vi "Grid_multiGrid.vi"() -> ()   [LabVIEW 2014]
uses:
  <userlib>/Nanonis Prog Interface V5/Nanonis Prog Interface.lvlib
panel:
  out "size(s) 5":i32
  out "size(s) 4":i32
  out "size(s) 3":i32=11
  out "size(s) 2":i32=12
  out "size(s)":i32=15
  out "data\n\n 5":T1(array[cluster])=[{"Amplitude (mod. signal unit)"=0.0, "Lockin on/off status"=FALSE, "Backward sweep"=TRUE, "Number of points"=215, "Channels"=["Current (A)", "LI Demod 1 X (A)", "LI Demod 1 Y (A)", "LI Demod 2 X (A)", "LI Demod 2 Y (A)"], "Parameters"=["X (m)", "Y (m)", "Z (m)", "Z offset (m)", "Settling time (s)", "Integration time (s)", "Z-Ctrl hold", "Final Z (m)"], "Fixed parameters"=["Sweep Start", "Sweep End"], "Multiple sweeps configuration"={"Number of Sweeps"=1, "Save all"=FALSE}, "Initialization"={"Z averaging time (s)"=0.001, "Initial settling time (s)"=0.0002}, "Sweep Timing"={"Max. slew rate (V/s)"=inf, "Settling time (s)"=0.001, "Integration time (s)"=0.001}, "End of Sweep"={"End settling time (s)"=5e-05, "Z control time (s)"=0.0002}, "Initial Z-Offset (m)"=0.0, "Sweep Distance (m)"=0.0, "Channels 2"=[], "Name"="", "Reset Z"=FALSE, "Record final Z"=FALSE, "Auto Retract Status"=FALSE, "Threshold"=0.0, "Auto Retract Signal Index"=0, "Auto Retract Condition"=FALSE}, {"Amplitude (mod. signal unit)"=0.0, "Lockin on/off status"=FALSE, "Backward sweep"=FALSE, "Number of points"=0, "Channels"=[], "Parameters"=[], "Fixed parameters"=[], "Multiple sweeps configuration"={"Number of Sweeps"=0, "Save all"=FALSE}, "Initialization"={"Z averaging time (s)"=0.0, "Initial settling time (s)"=0.0}, "Sweep Timing"={"Max. slew rate (V/s)"=0.0, "Settling time (s)"=0.0, "Integration time (s)"=0.0}, "End of Sweep"={"End settling time (s)"=0.0, "Z control time (s)"=0.0}, "Initial Z-Offset (m)"=0.0, "Sweep Distance (m)"=0.0, "Channels 2"=[], "Name"="", "Reset Z"=FALSE, "Record final Z"=FALSE, "Auto Retract Status"=FALSE, "Threshold"=0.0, "Auto Retract Signal Index"=0, "Auto Retract Condition"=FALSE}, {"Amplitude (mod. signal unit)"=0.0, "Lockin on/off status"=FALSE, "Backward sweep"=FALSE, "Number of points"=0, "Channels"=[], "Parameters"=[], "Fixed parameters"=[], "Multiple sweeps configuration"={"Number of Sweeps"=0, "Save all"=FALSE}, "Initialization"={"Z averaging time (s)"=0.0, "Initial settling time (s)"=0.0}, "Sweep Timing"={"Max. slew rate (V/s)"=0.0, "Settling time (s)"=0.0, "Integration time (s)"=0.0}, "End of Sweep"={"End settling time (s)"=0.0, "Z control time (s)"=0.0}, "Initial Z-Offset (m)"=0.0, "Sweep Distance (m)"=0.0, "Channels 2"=[], "Name"="", "Reset Z"=FALSE, "Record final Z"=FALSE, "Auto Retract Status"=FALSE, "Threshold"=0.0, "Auto Retract Signal Index"=0, "Auto Retract Condition"=FALSE}, {"Amplitude (mod. signal unit)"=0.0, "Lockin on/off status"=FALSE, "Backward sweep"=FALSE, "Number of points"=0, "Channels"=[], "Parameters"=[], "Fixed parameters"=[], "Multiple sweeps configuration"={"Number of Sweeps"=0, "Save all"=FALSE}, "Initialization"={"Z averaging time (s)"=0.0, "Initial settling time (s)"=0.0}, "Sweep Timing"={"Max. slew rate (V/s)"=0.0, "Settling time (s)"=0.0, "Integration time (s)"=0.0}, "End of Sweep"={"End settling time (s)"=0.0, "Z control time (s)"=0.0}, "Initial Z-Offset (m)"=0.0, "Sweep Distance (m)"=0.0, "Channels 2"=[], "Name"="", "Reset Z"=FALSE, "Record final Z"=FALSE, "Auto Retract Status"=FALSE, "Threshold"=0.0, "Auto Retract Signal Index"=0, "Auto Retract Condition"=FALSE}, {"Amplitude (mod. signal unit)"=0.0, "Lockin on/off status"=FALSE, "Backward sweep"=FALSE, "Number of points"=0, "Channels"=[], "Parameters"=[], "Fixed parameters"=[], "Multiple sweeps configuration"={"Number of Sweeps"=0, "Save all"=FALSE}, "Initialization"={"Z averaging time (s)"=0.0, "Initial settling time (s)"=0.0}, "Sweep Timing"={"Max. slew rate (V/s)"=0.0, "Settling time (s)"=0.0, "Integration time (s)"=0.0}, "End of Sweep"={"End settling time (s)"=0.0, "Z control time (s)"=0.0}, "Initial Z-Offset (m)"=0.0, "Sweep Distance (m)"=0.0, "Channels 2"=[], "Name"="", "Reset Z"=FALSE, "Record final Z"=FALSE, "Auto Retract Status"=FALSE, "Threshold"=0.0, "Auto Retract Signal Index"=0, "Auto Retract Condition"=FALSE}, {"Amplitude (mod. signal unit)"=0.0, "Lockin on/off status"=FALSE, "Backward sweep"=FALSE, "Number of points"=0, "Channels"=[], "Parameters"=[], "Fixed parameters"=[], "Multiple sweeps configuration"={"Number of Sweeps"=0, "Save all"=FALSE}, "Initialization"={"Z averaging time (s)"=0.0, "Initial settling time (s)"=0.0}, "Sweep Timing"={"Max. slew rate (V/s)"=0.0, "Settling time (s)"=0.0, "Integration time (s)"=0.0}, "End of Sweep"={"End settling time (s)"=0.0, "Z control time (s)"=0.0}, "Initial Z-Offset (m)"=0.0, "Sweep Distance (m)"=0.0, "Channels 2"=[], "Name"="", "Reset Z"=FALSE, "Record final Z"=FALSE, "Auto Retract Status"=FALSE, "Threshold"=0.0, "Auto Retract Signal Index"=0, "Auto Retract Condition"=FALSE}, {"Amplitude (mod. signal unit)"=0.0, "Lockin on/off status"=FALSE, "Backward sweep"=FALSE, "Number of points"=0, "Channels"=[], "Parameters"=[], "Fixed parameters"=[], "Multiple sweeps configuration"={"Number of Sweeps"=0, "Save all"=FALSE}, "Initialization"={"Z averaging time (s)"=0.0, "Initial settling time (s)"=0.0}, "Sweep Timing"={"Max. slew rate (V/s)"=0.0, "Settling time (s)"=0.0, "Integration time (s)"=0.0}, "End of Sweep"={"End settling time (s)"=0.0, "Z control time (s)"=0.0}, "Initial Z-Offset (m)"=0.0, "Sweep Distance (m)"=0.0, "Channels 2"=[], "Name"="", "Reset Z"=FALSE, "Record final Z"=FALSE, "Auto Retract Status"=FALSE, "Threshold"=0.0, "Auto Retract Signal Index"=0, "Auto Retract Condition"=FALSE}, {"Amplitude (mod. signal unit)"=0.0, "Lockin on/off status"=FALSE, "Backward sweep"=FALSE, "Number of points"=0, "Channels"=[], "Parameters"=[], "Fixed parameters"=[], "Multiple sweeps configuration"={"Number of Sweeps"=0, "Save all"=FALSE}, "Initialization"={"Z averaging time (s)"=0.0, "Initial settling time (s)"=0.0}, "Sweep Timing"={"Max. slew rate (V/s)"=0.0, "Settling time (s)"=0.0, "Integration time (s)"=0.0}, "End of Sweep"={"End settling time (s)"=0.0, "Z control time (s)"=0.0}, "Initial Z-Offset (m)"=0.0, "Sweep Distance (m)"=0.0, "Channels 2"=[], "Name"="", "Reset Z"=FALSE, "Record final Z"=FALSE, "Auto Retract Status"=FALSE, "Threshold"=0.0, "Auto Retract Signal Index"=0, "Auto Retract Condition"=FALSE}, {"Amplitude (mod. signal unit)"=0.0, "Lockin on/off status"=FALSE, "Backward sweep"=FALSE, "Number of points"=0, "Channels"=[], "Parameters"=[], "Fixed parameters"=[], "Multiple sweeps configuration"={"Number of Sweeps"=0, "Save all"=FALSE}, "Initialization"={"Z averaging time (s)"=0.0, "Initial settling time (s)"=0.0}, "Sweep Timing"={"Max. slew rate (V/s)"=0.0, "Settling time (s)"=0.0, "Integration time (s)"=0.0}, "End of Sweep"={"End settling time (s)"=0.0, "Z control time (s)"=0.0}, "Initial Z-Offset (m)"=0.0, "Sweep Distance (m)"=0.0, "Channels 2"=[], "Name"="", "Reset Z"=FALSE, "Record final Z"=FALSE, "Auto Retract Status"=FALSE, "Threshold"=0.0, "Auto Retract Signal Index"=0, "Auto Retract Condition"=FALSE}, {"Amplitude (mod. signal unit)"=0.0, "Lockin on/off status"=FALSE, "Backward sweep"=FALSE, "Number of points"=0, "Channels"=[], "Parameters"=[], "Fixed parameters"=[], "Multiple sweeps configuration"={"Number of Sweeps"=0, "Save all"=FALSE}, "Initialization"={"Z averaging time (s)"=0.0, "Initial settling time (s)"=0.0}, "Sweep Timing"={"Max. slew rate (V/s)"=0.0, "Settling time (s)"=0.0, "Integration time (s)"=0.0}, "End of Sweep"={"End settling time (s)"=0.0, "Z control time (s)"=0.0}, "Initial Z-Offset (m)"=0.0, "Sweep Distance (m)"=0.0, "Channels 2"=[], "Name"="", "Reset Z"=FALSE, "Record final Z"=FALSE, "Auto Retract Status"=FALSE, "Threshold"=0.0, "Auto Retract Signal Index"=0, "Auto Retract Condition"=FALSE}, {"Amplitude (mod. signal unit)"=0.0, "Lockin on/off status"=FALSE, "Backward sweep"=FALSE, "Number of points"=0, "Channels"=[], "Parameters"=[], "Fixed parameters"=[], "Multiple sweeps configuration"={"Number of Sweeps"=0, "Save all"=FALSE}, "Initialization"={"Z averaging time (s)"=0.0, "Initial settling time (s)"=0.0}, "Sweep Timing"={"Max. slew rate (V/s)"=0.0, "Settling time (s)"=0.0, "Integration time (s)"=0.0}, "End of Sweep"={"End settling time (s)"=0.0, "Z control time (s)"=0.0}, "Initial Z-Offset (m)"=0.0, "Sweep Distance (m)"=0.0, "Channels 2"=[], "Name"="", "Reset Z"=FALSE, "Record final Z"=FALSE, "Auto Retract Status"=FALSE, "Threshold"=0.0, "Auto Retract Signal Index"=0, "Auto Retract Condition"=FALSE}, {"Amplitude (mod. signal unit)"=0.0, "Lockin on/off status"=FALSE, "Backward sweep"=FALSE, "Number of points"=0, "Channels"=[], "Parameters"=[], "Fixed parameters"=[], "Multiple sweeps configuration"={"Number of Sweeps"=0, "Save all"=FALSE}, "Initialization"={"Z averaging time (s)"=0.0, "Initial settling time (s)"=0.0}, "Sweep Timing"={"Max. slew rate (V/s)"=0.0, "Settling time (s)"=0.0, "Integration time (s)"=0.0}, "End of Sweep"={"End settling time (s)"=0.0, "Z control time (s)"=0.0}, "Initial Z-Offset (m)"=0.0, "Sweep Distance (m)"=0.0, "Channels 2"=[], "Name"="", "Reset Z"=FALSE, "Record final Z"=FALSE, "Auto Retract Status"=FALSE, "Threshold"=0.0, "Auto Retract Signal Index"=0, "Auto Retract Condition"=FALSE}, {"Amplitude (mod. signal unit)"=0.0, "Lockin on/off status"=FALSE, "Backward sweep"=FALSE, "Number of points"=0, "Channels"=[], "Parameters"=[], "Fixed parameters"=[], "Multiple sweeps configuration"={"Number of Sweeps"=0, "Save all"=FALSE}, "Initialization"={"Z averaging time (s)"=0.0, "Initial settling time (s)"=0.0}, "Sweep Timing"={"Max. slew rate (V/s)"=0.0, "Settling time (s)"=0.0, "Integration time (s)"=0.0}, "End of Sweep"={"End settling time (s)"=0.0, "Z control time (s)"=0.0}, "Initial Z-Offset (m)"=0.0, "Sweep Distance (m)"=0.0, "Channels 2"=[], "Name"="", "Reset Z"=FALSE, "Record final Z"=FALSE, "Auto Retract Status"=FALSE, "Threshold"=0.0, "Auto Retract Signal Index"=0, "Auto Retract Condition"=FALSE}, {"Amplitude (mod. signal unit)"=0.0, "Lockin on/off status"=FALSE, "Backward sweep"=FALSE, "Number of points"=0, "Channels"=[], "Parameters"=[], "Fixed parameters"=[], "Multiple sweeps configuration"={"Number of Sweeps"=0, "Save all"=FALSE}, "Initialization"={"Z averaging time (s)"=0.0, "Initial settling time (s)"=0.0}, "Sweep Timing"={"Max. slew rate (V/s)"=0.0, "Settling time (s)"=0.0, "Integration time (s)"=0.0}, "End of Sweep"={"End settling time (s)"=0.0, "Z control time (s)"=0.0}, "Initial Z-Offset (m)"=0.0, "Sweep Distance (m)"=0.0, "Channels 2"=[], "Name"="", "Reset Z"=FALSE, "Record final Z"=FALSE, "Auto Retract Status"=FALSE, "Threshold"=0.0, "Auto Retract Signal Index"=0, "Auto Retract Condition"=FALSE}, {"Amplitude (mod. signal unit)"=0.0, "Lockin on/off status"=FALSE, "Backward sweep"=FALSE, "Number of points"=0, "Channels"=[], "Parameters"=[], "Fixed parameters"=[], "Multiple sweeps configuration"={"Number of Sweeps"=0, "Save all"=FALSE}, "Initialization"={"Z averaging time (s)"=0.0, "Initial settling time (s)"=0.0}, "Sweep Timing"={"Max. slew rate (V/s)"=0.0, "Settling time (s)"=0.0, "Integration time (s)"=0.0}, "End of Sweep"={"End settling time (s)"=0.0, "Z control time (s)"=0.0}, "Initial Z-Offset (m)"=0.0, "Sweep Distance (m)"=0.0, "Channels 2"=[], "Name"="", "Reset Z"=FALSE, "Record final Z"=FALSE, "Auto Retract Status"=FALSE, "Threshold"=0.0, "Auto Retract Signal Index"=0, "Auto Retract Condition"=FALSE}, {"Amplitude (mod. signal unit)"=0.0, "Lockin on/off status"=FALSE, "Backward sweep"=FALSE, "Number of points"=0, "Channels"=[], "Parameters"=[], "Fixed parameters"=[], "Multiple sweeps configuration"={"Number of Sweeps"=0, "Save all"=FALSE}, "Initialization"={"Z averaging time (s)"=0.0, "Initial settling time (s)"=0.0}, "Sweep Timing"={"Max. slew rate (V/s)"=0.0, "Settling time (s)"=0.0, "Integration time (s)"=0.0}, "End of Sweep"={"End settling time (s)"=0.0, "Z control time (s)"=0.0}, "Initial Z-Offset (m)"=0.0, "Sweep Distance (m)"=0.0, "Channels 2"=[], "Name"="", "Reset Z"=FALSE, "Record final Z"=FALSE, "Auto Retract Status"=FALSE, "Threshold"=0.0, "Auto Retract Signal Index"=0, "Auto Retract Condition"=FALSE}, {"Amplitude (mod. signal unit)"=0.0, "Lockin on/off status"=FALSE, "Backward sweep"=FALSE, "Number of points"=0, "Channels"=[], "Parameters"=[], "Fixed parameters"=[], "Multiple sweeps configuration"={"Number of Sweeps"=0, "Save all"=FALSE}, "Initialization"={"Z averaging time (s)"=0.0, "Initial settling time (s)"=0.0}, "Sweep Timing"={"Max. slew rate (V/s)"=0.0, "Settling time (s)"=0.0, "Integration time (s)"=0.0}, "End of Sweep"={"End settling time (s)"=0.0, "Z control time (s)"=0.0}, "Initial Z-Offset (m)"=0.0, "Sweep Distance (m)"=0.0, "Channels 2"=[], "Name"="", "Reset Z"=FALSE, "Record final Z"=FALSE, "Auto Retract Status"=FALSE, "Threshold"=0.0, "Auto Retract Signal Index"=0, "Auto Retract Condition"=FALSE}, {"Amplitude (mod. signal unit)"=0.0, "Lockin on/off status"=FALSE, "Backward sweep"=FALSE, "Number of points"=0, "Channels"=[], "Parameters"=[], "Fixed parameters"=[], "Multiple sweeps configuration"={"Number of Sweeps"=0, "Save all"=FALSE}, "Initialization"={"Z averaging time (s)"=0.0, "Initial settling time (s)"=0.0}, "Sweep Timing"={"Max. slew rate (V/s)"=0.0, "Settling time (s)"=0.0, "Integration time (s)"=0.0}, "End of Sweep"={"End settling time (s)"=0.0, "Z control time (s)"=0.0}, "Initial Z-Offset (m)"=0.0, "Sweep Distance (m)"=0.0, "Channels 2"=[], "Name"="", "Reset Z"=FALSE, "Record final Z"=FALSE, "Auto Retract Status"=FALSE, "Threshold"=0.0, "Auto Retract Signal Index"=0, "Auto Retract Condition"=FALSE}]
  out "data\n\n 2":T2(array[cluster])=[{"Amplitude (mod. signal unit)"=0.0, "Lockin on/off status"=FALSE, "Advanced options"={"Z-Controller Hold"=TRUE, "Record final Z"=FALSE, "Reset Bias"=TRUE}, "Backward sweep"=TRUE, "Number of points"=215, "Channels"=["Current (A)", "LI Demod 1 X (A)", "LI Demod 1 Y (A)", "LI Demod 2 X (A)", "LI Demod 2 Y (A)"], "Parameters"=["X (m)", "Y (m)", "Z (m)", "Z offset (m)", "Settling time (s)", "Integration time (s)", "Z-Ctrl hold", "Final Z (m)"], "Fixed parameters"=["Sweep Start", "Sweep End"], "Multiple sweeps configuration"={"Number of Sweeps"=1, "Save all"=FALSE}, "Initialization"={"Z averaging time (s)"=0.001, "Z offset (m)"=0.0, "Initial settling time (s)"=0.0002}, "Sweep Timing"={"Max. slew rate (V/s)"=inf, "Settling time (s)"=0.001, "Integration time (s)"=0.001}, "End of Sweep"={"End settling time (s)"=5e-05, "Z control time (s)"=0.0002}, "Start value (V)"=-0.02, "End value (V)"=-3.0, "Channels 2"=[0, 20, 21, 22, 23], "Name"="numerical_DCA_-20mV->-3V"}, {"Amplitude (mod. signal unit)"=0.0, "Lockin on/off status"=FALSE, "Advanced options"={"Z-Controller Hold"=TRUE, "Record final Z"=FALSE, "Reset Bias"=TRUE}, "Backward sweep"=TRUE, "Number of points"=215, "Channels"=["Current (A)", "LI Demod 1 X (A)", "LI Demod 1 Y (A)", "LI Demod 2 X (A)", "LI Demod 2 Y (A)"], "Parameters"=["X (m)", "Y (m)", "Z (m)", "Z offset (m)", "Settling time (s)", "Integration time (s)", "Z-Ctrl hold", "Final Z (m)"], "Fixed parameters"=["Sweep Start", "Sweep End"], "Multiple sweeps configuration"={"Number of Sweeps"=1, "Save all"=FALSE}, "Initialization"={"Z averaging time (s)"=0.001, "Z offset (m)"=0.0, "Initial settling time (s)"=0.0002}, "Sweep Timing"={"Max. slew rate (V/s)"=inf, "Settling time (s)"=0.001, "Integration time (s)"=0.001}, "End of Sweep"={"End settling time (s)"=5e-05, "Z control time (s)"=0.0002}, "Start value (V)"=-0.02, "End value (V)"=0.7, "Channels 2"=[0, 20, 21, 22, 23], "Name"="numerical_DCA_-20mV->0.7V"}, {"Amplitude (mod. signal unit)"=0.0, "Lockin on/off status"=FALSE, "Advanced options"={"Z-Controller Hold"=TRUE, "Record final Z"=FALSE, "Reset Bias"=TRUE}, "Backward sweep"=TRUE, "Number of points"=215, "Channels"=["Current (A)", "LI Demod 1 X (A)", "LI Demod 1 Y (A)", "LI Demod 2 X (A)", "LI Demod 2 Y (A)"], "Parameters"=["X (m)", "Y (m)", "Z (m)", "Z offset (m)", "Settling time (s)", "Integration time (s)", "Z-Ctrl hold", "Final Z (m)"], "Fixed parameters"=["Sweep Start", "Sweep End"], "Multiple sweeps configuration"={"Number of Sweeps"=30, "Save all"=FALSE}, "Initialization"={"Z averaging time (s)"=0.001, "Z offset (m)"=0.0, "Initial settling time (s)"=0.0002}, "Sweep Timing"={"Max. slew rate (V/s)"=inf, "Settling time (s)"=0.001, "Integration time (s)"=0.001}, "End of Sweep"={"End settling time (s)"=5e-05, "Z control time (s)"=0.0002}, "Start value (V)"=-0.02, "End value (V)"=0.7, "Channels 2"=[0, 20, 21, 22, 23], "Name"="numerical_DCA_-20mV->-0.7V_30sweeps"}, {"Amplitude (mod. signal unit)"=0.0, "Lockin on/off status"=FALSE, "Advanced options"={"Z-Controller Hold"=TRUE, "Record final Z"=FALSE, "Reset Bias"=TRUE}, "Backward sweep"=TRUE, "Number of points"=215, "Channels"=["Current (A)", "LI Demod 1 X (A)", "LI Demod 1 Y (A)", "LI Demod 2 X (A)", "LI Demod 2 Y (A)"], "Parameters"=["X (m)", "Y (m)", "Z (m)", "Z offset (m)", "Settling time (s)", "Integration time (s)", "Z-Ctrl hold", "Final Z (m)"], "Fixed parameters"=["Sweep Start", "Sweep End"], "Multiple sweeps configuration"={"Number of Sweeps"=50, "Save all"=FALSE}, "Initialization"={"Z averaging time (s)"=0.001, "Z offset (m)"=0.0, "Initial settling time (s)"=0.0002}, "Sweep Timing"={"Max. slew rate (V/s)"=inf, "Settling time (s)"=0.001, "Integration time (s)"=0.001}, "End of Sweep"={"End settling time (s)"=5e-05, "Z control time (s)"=0.0002}, "Start value (V)"=-0.02, "End value (V)"=0.7, "Channels 2"=[0, 20, 21, 22, 23], "Name"="numerical_DCA_-20mV->-0.7V_50_sweeps"}, {"Amplitude (mod. signal unit)"=0.0, "Lockin on/off status"=FALSE, "Advanced options"={"Z-Controller Hold"=TRUE, "Record final Z"=FALSE, "Reset Bias"=TRUE}, "Backward sweep"=TRUE, "Number of points"=215, "Channels"=["Current (A)", "LI Demod 1 X (A)", "LI Demod 1 Y (A)", "LI Demod 2 X (A)", "LI Demod 2 Y (A)"], "Parameters"=["X (m)", "Y (m)", "Z (m)", "Z offset (m)", "Settling time (s)", "Integration time (s)", "Z-Ctrl hold", "Final Z (m)"], "Fixed parameters"=["Sweep Start", "Sweep End"], "Multiple sweeps configuration"={"Number of Sweeps"=70, "Save all"=FALSE}, "Initialization"={"Z averaging time (s)"=0.001, "Z offset (m)"=0.0, "Initial settling time (s)"=0.0002}, "Sweep Timing"={"Max. slew rate (V/s)"=inf, "Settling time (s)"=0.001, "Integration time (s)"=0.001}, "End of Sweep"={"End settling time (s)"=5e-05, "Z control time (s)"=0.0002}, "Start value (V)"=-0.02, "End value (V)"=-3.0, "Channels 2"=[0, 20, 21, 22, 23], "Name"="numerical_DCA_-20mV->-3V_70sweeps"}, {"Amplitude (mod. signal unit)"=0.0, "Lockin on/off status"=FALSE, "Advanced options"={"Z-Controller Hold"=TRUE, "Record final Z"=FALSE, "Reset Bias"=TRUE}, "Backward sweep"=TRUE, "Number of points"=215, "Channels"=["Current (A)", "LI Demod 1 X (A)", "LI Demod 1 Y (A)", "LI Demod 2 X (A)", "LI Demod 2 Y (A)"], "Parameters"=["X (m)", "Y (m)", "Z (m)", "Z offset (m)", "Settling time (s)", "Integration time (s)", "Z-Ctrl hold", "Final Z (m)"], "Fixed parameters"=["Sweep Start", "Sweep End"], "Multiple sweeps configuration"={"Number of Sweeps"=100, "Save all"=FALSE}, "Initialization"={"Z averaging time (s)"=0.001, "Z offset (m)"=0.0, "Initial settling time (s)"=0.0002}, "Sweep Timing"={"Max. slew rate (V/s)"=inf, "Settling time (s)"=0.001, "Integration time (s)"=0.001}, "End of Sweep"={"End settling time (s)"=5e-05, "Z control time (s)"=0.0002}, "Start value (V)"=-0.02, "End value (V)"=-3.0, "Channels 2"=[0, 20, 21, 22, 23], "Name"="numerical_DCA_-20mV->3V_100_sweeps"}, {"Amplitude (mod. signal unit)"=0.0, "Lockin on/off status"=FALSE, "Advanced options"={"Z-Controller Hold"=TRUE, "Record final Z"=FALSE, "Reset Bias"=TRUE}, "Backward sweep"=TRUE, "Number of points"=256, "Channels"=["Current (A)", "LI Demod 1 X (A)", "LI Demod 1 Y (A)", "LI Demod 2 X (A)", "LI Demod 2 Y (A)"], "Parameters"=["X (m)", "Y (m)", "Z (m)", "Z offset (m)", "Settling time (s)", "Integration time (s)", "Z-Ctrl hold", "Final Z (m)"], "Fixed parameters"=["Sweep Start", "Sweep End"], "Multiple sweeps configuration"={"Number of Sweeps"=100, "Save all"=FALSE}, "Initialization"={"Z averaging time (s)"=0.001, "Z offset (m)"=0.0, "Initial settling time (s)"=5e-05}, "Sweep Timing"={"Max. slew rate (V/s)"=inf, "Settling time (s)"=0.001, "Integration time (s)"=0.0005}, "End of Sweep"={"End settling time (s)"=5e-05, "Z control time (s)"=5e-05}, "Start value (V)"=-1.0, "End value (V)"=2.0, "Channels 2"=[0, 20, 21, 22, 23], "Name"="numerical_-1V->2V"}, {"Amplitude (mod. signal unit)"=0.0, "Lockin on/off status"=FALSE, "Advanced options"={"Z-Controller Hold"=TRUE, "Record final Z"=FALSE, "Reset Bias"=TRUE}, "Backward sweep"=TRUE, "Number of points"=256, "Channels"=["Current (A)", "LI Demod 1 X (A)", "LI Demod 1 Y (A)", "LI Demod 2 X (A)", "LI Demod 2 Y (A)"], "Parameters"=["X (m)", "Y (m)", "Z (m)", "Z offset (m)", "Settling time (s)", "Integration time (s)", "Z-Ctrl hold", "Final Z (m)"], "Fixed parameters"=["Sweep Start", "Sweep End"], "Multiple sweeps configuration"={"Number of Sweeps"=100, "Save all"=FALSE}, "Initialization"={"Z averaging time (s)"=0.001, "Z offset (m)"=0.0, "Initial settling time (s)"=5e-05}, "Sweep Timing"={"Max. slew rate (V/s)"=inf, "Settling time (s)"=0.001, "Integration time (s)"=0.0005}, "End of Sweep"={"End settling time (s)"=5e-05, "Z control time (s)"=5e-05}, "Start value (V)"=-0.02, "End value (V)"=0.02, "Channels 2"=[0, 20, 21, 22, 23], "Name"="numerical_-20mV->20mV"}, {"Amplitude (mod. signal unit)"=0.0, "Lockin on/off status"=FALSE, "Advanced options"={"Z-Controller Hold"=TRUE, "Record final Z"=FALSE, "Reset Bias"=TRUE}, "Backward sweep"=TRUE, "Number of points"=286, "Channels"=["Current (A)", "LI Demod 1 X (A)", "LI Demod 1 Y (A)", "LI Demod 2 X (A)", "LI Demod 2 Y (A)"], "Parameters"=["X (m)", "Y (m)", "Z (m)", "Z offset (m)", "Settling time (s)", "Integration time (s)", "Z-Ctrl hold", "Final Z (m)"], "Fixed parameters"=["Sweep Start", "Sweep End"], "Multiple sweeps configuration"={"Number of Sweeps"=50, "Save all"=FALSE}, "Initialization"={"Z averaging time (s)"=0.001, "Z offset (m)"=0.0, "Initial settling time (s)"=5e-05}, "Sweep Timing"={"Max. slew rate (V/s)"=inf, "Settling time (s)"=0.001, "Integration time (s)"=0.0005}, "End of Sweep"={"End settling time (s)"=5e-05, "Z control time (s)"=5e-05}, "Start value (V)"=-0.2, "End value (V)"=0.8, "Channels 2"=[0, 20, 21, 22, 23], "Name"="DCA_numerical_-0.2V->0.8V"}, {"Amplitude (mod. signal unit)"=0.0, "Lockin on/off status"=FALSE, "Advanced options"={"Z-Controller Hold"=TRUE, "Record final Z"=FALSE, "Reset Bias"=TRUE}, "Backward sweep"=TRUE, "Number of points"=421, "Channels"=["Current (A)", "LI Demod 1 X (A)", "LI Demod 1 Y (A)", "LI Demod 2 X (A)", "LI Demod 2 Y (A)"], "Parameters"=["X (m)", "Y (m)", "Z (m)", "Z offset (m)", "Settling time (s)", "Integration time (s)", "Z-Ctrl hold", "Final Z (m)"], "Fixed parameters"=["Sweep Start", "Sweep End"], "Multiple sweeps configuration"={"Number of Sweeps"=100, "Save all"=FALSE}, "Initialization"={"Z averaging time (s)"=0.001, "Z offset (m)"=0.0, "Initial settling time (s)"=5e-05}, "Sweep Timing"={"Max. slew rate (V/s)"=inf, "Settling time (s)"=0.001, "Integration time (s)"=0.0005}, "End of Sweep"={"End settling time (s)"=5e-05, "Z control time (s)"=5e-05}, "Start value (V)"=-2.0, "End value (V)"=2.2, "Channels 2"=[0, 20, 21, 22, 23], "Name"="numerical_-2V->2.2V"}, {"Amplitude (mod. signal unit)"=0.0, "Lockin on/off status"=FALSE, "Advanced options"={"Z-Controller Hold"=TRUE, "Record final Z"=FALSE, "Reset Bias"=TRUE}, "Backward sweep"=TRUE, "Number of points"=500, "Channels"=["Current (A)", "LI Demod 1 X (A)", "LI Demod 1 Y (A)", "LI Demod 2 X (A)", "LI Demod 2 Y (A)"], "Parameters"=["X (m)", "Y (m)", "Z (m)", "Z offset (m)", "Settling time (s)", "Integration time (s)", "Z-Ctrl hold", "Final Z (m)"], "Fixed parameters"=["Sweep Start", "Sweep End"], "Multiple sweeps configuration"={"Number of Sweeps"=20, "Save all"=FALSE}, "Initialization"={"Z averaging time (s)"=0.001, "Z offset (m)"=0.0, "Initial settling time (s)"=0.01}, "Sweep Timing"={"Max. slew rate (V/s)"=inf, "Settling time (s)"=0.001, "Integration time (s)"=0.001}, "End of Sweep"={"End settling time (s)"=0.1, "Z control time (s)"=0.001}, "Start value (V)"=-0.2, "End value (V)"=0.8, "Channels 2"=[0, 20, 21, 22, 23], "Name"="DCA_numerical2_-0.2V->0.8V"}, {"Amplitude (mod. signal unit)"=0.0015, "Lockin on/off status"=FALSE, "Advanced options"={"Z-Controller Hold"=TRUE, "Record final Z"=FALSE, "Reset Bias"=TRUE}, "Backward sweep"=TRUE, "Number of points"=80, "Channels"=["Current (A)", "LI Demod 1 X (A)", "LI Demod 1 Y (A)", "LI Demod 2 X (A)", "LI Demod 2 Y (A)"], "Parameters"=["X (m)", "Y (m)", "Z (m)", "Z offset (m)", "Settling time (s)", "Integration time (s)", "Z-Ctrl hold", "Final Z (m)"], "Fixed parameters"=["Sweep Start", "Sweep End"], "Multiple sweeps configuration"={"Number of Sweeps"=10, "Save all"=FALSE}, "Initialization"={"Z averaging time (s)"=0.001, "Z offset (m)"=0.0, "Initial settling time (s)"=0.0046}, "Sweep Timing"={"Max. slew rate (V/s)"=inf, "Settling time (s)"=0.0046, "Integration time (s)"=0.032}, "End of Sweep"={"End settling time (s)"=5e-05, "Z control time (s)"=5e-05}, "Start value (V)"=-0.02, "End value (V)"=0.02, "Channels 2"=[0, 20, 21, 22, 23], "Name"="lockin_-20mV->20mV"}, {"Amplitude (mod. signal unit)"=0.002, "Lockin on/off status"=FALSE, "Advanced options"={"Z-Controller Hold"=TRUE, "Record final Z"=FALSE, "Reset Bias"=TRUE}, "Backward sweep"=TRUE, "Number of points"=70, "Channels"=["Current (A)", "LI Demod 1 X (A)", "LI Demod 1 Y (A)", "LI Demod 2 X (A)", "LI Demod 2 Y (A)"], "Parameters"=["X (m)", "Y (m)", "Z (m)", "Z offset (m)", "Settling time (s)", "Integration time (s)", "Z-Ctrl hold", "Final Z (m)"], "Fixed parameters"=["Sweep Start", "Sweep End"], "Multiple sweeps configuration"={"Number of Sweeps"=10, "Save all"=FALSE}, "Initialization"={"Z averaging time (s)"=0.001, "Z offset (m)"=0.0, "Initial settling time (s)"=0.0046}, "Sweep Timing"={"Max. slew rate (V/s)"=inf, "Settling time (s)"=0.0046, "Integration time (s)"=0.032}, "End of Sweep"={"End settling time (s)"=5e-05, "Z control time (s)"=5e-05}, "Start value (V)"=-0.025, "End value (V)"=0.025, "Channels 2"=[0, 20, 21, 22, 23], "Name"="lockin_-25mV->25mV"}, {"Amplitude (mod. signal unit)"=0.002, "Lockin on/off status"=FALSE, "Advanced options"={"Z-Controller Hold"=TRUE, "Record final Z"=FALSE, "Reset Bias"=TRUE}, "Backward sweep"=TRUE, "Number of points"=70, "Channels"=["Current (A)", "LI Demod 1 X (A)", "LI Demod 1 Y (A)", "LI Demod 2 X (A)", "LI Demod 2 Y (A)"], "Parameters"=["X (m)", "Y (m)", "Z (m)", "Z offset (m)", "Settling time (s)", "Integration time (s)", "Z-Ctrl hold", "Final Z (m)"], "Fixed parameters"=["Sweep Start", "Sweep End"], "Multiple sweeps configuration"={"Number of Sweeps"=10, "Save all"=FALSE}, "Initialization"={"Z averaging time (s)"=0.001, "Z offset (m)"=0.0, "Initial settling time (s)"=0.0046}, "Sweep Timing"={"Max. slew rate (V/s)"=inf, "Settling time (s)"=0.0046, "Integration time (s)"=0.032}, "End of Sweep"={"End settling time (s)"=5e-05, "Z control time (s)"=5e-05}, "Start value (V)"=-0.025, "End value (V)"=0.025, "Channels 2"=[0, 20, 21, 22, 23], "Name"="test"}, {"Amplitude (mod. signal unit)"=0.0025, "Lockin on/off status"=FALSE, "Advanced options"={"Z-Controller Hold"=TRUE, "Record final Z"=FALSE, "Reset Bias"=TRUE}, "Backward sweep"=TRUE, "Number of points"=320, "Channels"=["Current (A)", "LI Demod 1 X (A)", "LI Demod 1 Y (A)", "LI Demod 2 X (A)", "LI Demod 2 Y (A)"], "Parameters"=["X (m)", "Y (m)", "Z (m)", "Z offset (m)", "Settling time (s)", "Integration time (s)", "Z-Ctrl hold", "Final Z (m)"], "Fixed parameters"=["Sweep Start", "Sweep End"], "Multiple sweeps configuration"={"Number of Sweeps"=1, "Save all"=FALSE}, "Initialization"={"Z averaging time (s)"=0.001, "Z offset (m)"=0.0, "Initial settling time (s)"=0.0046}, "Sweep Timing"={"Max. slew rate (V/s)"=inf, "Settling time (s)"=0.0046, "Integration time (s)"=0.0042}, "End of Sweep"={"End settling time (s)"=5e-05, "Z control time (s)"=5e-05}, "Start value (V)"=0.02, "End value (V)"=-0.02, "Channels 2"=[0, 20, 21, 22, 23], "Name"="lockin_highRes_20mV_-20mV"}, {"Amplitude (mod. signal unit)"=0.005, "Lockin on/off status"=FALSE, "Advanced options"={"Z-Controller Hold"=TRUE, "Record final Z"=FALSE, "Reset Bias"=TRUE}, "Backward sweep"=TRUE, "Number of points"=256, "Channels"=["Current (A)", "LI Demod 1 X (A)", "LI Demod 1 Y (A)", "LI Demod 2 X (A)", "LI Demod 2 Y (A)"], "Parameters"=["X (m)", "Y (m)", "Z (m)", "Z offset (m)", "Settling time (s)", "Integration time (s)", "Z-Ctrl hold", "Final Z (m)"], "Fixed parameters"=["Sweep Start", "Sweep End"], "Multiple sweeps configuration"={"Number of Sweeps"=2, "Save all"=FALSE}, "Initialization"={"Z averaging time (s)"=0.001, "Z offset (m)"=0.0, "Initial settling time (s)"=0.0033}, "Sweep Timing"={"Max. slew rate (V/s)"=inf, "Settling time (s)"=0.0033, "Integration time (s)"=0.0164}, "End of Sweep"={"End settling time (s)"=5e-05, "Z control time (s)"=5e-05}, "Start value (V)"=-1.0, "End value (V)"=2.0, "Channels 2"=[0, 20, 21, 22, 23], "Name"="lockin_slow"}, {"Amplitude (mod. signal unit)"=0.005, "Lockin on/off status"=FALSE, "Advanced options"={"Z-Controller Hold"=TRUE, "Record final Z"=FALSE, "Reset Bias"=TRUE}, "Backward sweep"=TRUE, "Number of points"=310, "Channels"=["Current (A)", "LI Demod 1 X (A)", "LI Demod 1 Y (A)", "LI Demod 2 X (A)", "LI Demod 2 Y (A)"], "Parameters"=["X (m)", "Y (m)", "Z (m)", "Z offset (m)", "Settling time (s)", "Integration time (s)", "Z-Ctrl hold", "Final Z (m)"], "Fixed parameters"=["Sweep Start", "Sweep End"], "Multiple sweeps configuration"={"Number of Sweeps"=2, "Save all"=FALSE}, "Initialization"={"Z averaging time (s)"=0.001, "Z offset (m)"=0.0, "Initial settling time (s)"=0.0031}, "Sweep Timing"={"Max. slew rate (V/s)"=inf, "Settling time (s)"=0.0031, "Integration time (s)"=0.0246}, "End of Sweep"={"End settling time (s)"=5e-05, "Z control time (s)"=5e-05}, "Start value (V)"=1.5, "End value (V)"=-0.05, "Channels 2"=[0, 20, 21, 22, 23], "Name"="Lock_in_DCA_1.5V->-50mV"}, {"Amplitude (mod. signal unit)"=0.005, "Lockin on/off status"=FALSE, "Advanced options"={"Z-Controller Hold"=TRUE, "Record final Z"=FALSE, "Reset Bias"=TRUE}, "Backward sweep"=TRUE, "Number of points"=401, "Channels"=["Current (A)", "Z (m)", "LI Demod 1 X (A)", "LI Demod 1 Y (A)", "LI Demod 2 X (A)", "LI Demod 2 Y (A)"], "Parameters"=["X (m)", "Y (m)", "Z (m)", "Z offset (m)", "Settling time (s)", "Integration time (s)", "Z-Ctrl hold", "Final Z (m)"], "Fixed parameters"=["Sweep Start", "Sweep End"], "Multiple sweeps configuration"={"Number of Sweeps"=1, "Save all"=FALSE}, "Initialization"={"Z averaging time (s)"=0.001, "Z offset (m)"=0.0, "Initial settling time (s)"=0.004}, "Sweep Timing"={"Max. slew rate (V/s)"=inf, "Settling time (s)"=0.02, "Integration time (s)"=0.015}, "End of Sweep"={"End settling time (s)"=5e-05, "Z control time (s)"=0.001}, "Start value (V)"=-1.0, "End value (V)"=1.0, "Channels 2"=[0, 14, 20, 21, 22, 23], "Name"="Long_MgPc_lockin_-1->1V"}, {"Amplitude (mod. signal unit)"=0.005, "Lockin on/off status"=FALSE, "Advanced options"={"Z-Controller Hold"=TRUE, "Record final Z"=FALSE, "Reset Bias"=TRUE}, "Backward sweep"=TRUE, "Number of points"=467, "Channels"=["Current (A)", "Z (m)", "LI Demod 1 X (A)", "LI Demod 1 Y (A)", "LI Demod 2 X (A)", "LI Demod 2 Y (A)"], "Parameters"=["X (m)", "Y (m)", "Z (m)", "Z offset (m)", "Settling time (s)", "Integration time (s)", "Z-Ctrl hold", "Final Z (m)"], "Fixed parameters"=["Sweep Start", "Sweep End"], "Multiple sweeps configuration"={"Number of Sweeps"=2, "Save all"=FALSE}, "Initialization"={"Z averaging time (s)"=0.001, "Z offset (m)"=0.0, "Initial settling time (s)"=0.004}, "Sweep Timing"={"Max. slew rate (V/s)"=inf, "Settling time (s)"=0.02, "Integration time (s)"=0.0246}, "End of Sweep"={"End settling time (s)"=5e-05, "Z control time (s)"=0.001}, "Start value (V)"=-2.0, "End value (V)"=1.5, "Channels 2"=[0, 14, 20, 21, 22, 23], "Name"="MgPc_long_lockin"}, {"Amplitude (mod. signal unit)"=0.008, "Lockin on/off status"=FALSE, "Advanced options"={"Z-Controller Hold"=TRUE, "Record final Z"=FALSE, "Reset Bias"=TRUE}, "Backward sweep"=TRUE, "Number of points"=256, "Channels"=["Current (A)", "LI Demod 1 X (A)", "LI Demod 1 Y (A)", "LI Demod 2 X (A)", "LI Demod 2 Y (A)"], "Parameters"=["X (m)", "Y (m)", "Z (m)", "Z offset (m)", "Settling time (s)", "Integration time (s)", "Z-Ctrl hold", "Final Z (m)"], "Fixed parameters"=["Sweep Start", "Sweep End"], "Multiple sweeps configuration"={"Number of Sweeps"=3, "Save all"=FALSE}, "Initialization"={"Z averaging time (s)"=0.001, "Z offset (m)"=0.0, "Initial settling time (s)"=0.0033}, "Sweep Timing"={"Max. slew rate (V/s)"=inf, "Settling time (s)"=0.0033, "Integration time (s)"=0.0082}, "End of Sweep"={"End settling time (s)"=5e-05, "Z control time (s)"=5e-05}, "Start value (V)"=-1.0, "End value (V)"=2.0, "Channels 2"=[0, 20, 21, 22, 23], "Name"="lockin_slow_-1_2"}, {"Amplitude (mod. signal unit)"=0.008, "Lockin on/off status"=FALSE, "Advanced options"={"Z-Controller Hold"=TRUE, "Record final Z"=FALSE, "Reset Bias"=TRUE}, "Backward sweep"=TRUE, "Number of points"=421, "Channels"=["Current (A)", "Z (m)", "LI Demod 1 X (A)", "LI Demod 1 Y (A)", "LI Demod 2 X (A)", "LI Demod 2 Y (A)"], "Parameters"=["X (m)", "Y (m)", "Z (m)", "Z offset (m)", "Settling time (s)", "Integration time (s)", "Z-Ctrl hold", "Final Z (m)"], "Fixed parameters"=["Sweep Start", "Sweep End"], "Multiple sweeps configuration"={"Number of Sweeps"=2, "Save all"=FALSE}, "Initialization"={"Z averaging time (s)"=0.001, "Z offset (m)"=0.0, "Initial settling time (s)"=5e-05}, "Sweep Timing"={"Max. slew rate (V/s)"=inf, "Settling time (s)"=0.0164, "Integration time (s)"=0.0164}, "End of Sweep"={"End settling time (s)"=5e-05, "Z control time (s)"=0.001}, "Start value (V)"=-2.0, "End value (V)"=2.2, "Channels 2"=[0, 14, 20, 21, 22, 23], "Name"="MgPc_long_lockin2"}, {"Amplitude (mod. signal unit)"=0.01, "Lockin on/off status"=FALSE, "Advanced options"={"Z-Controller Hold"=TRUE, "Record final Z"=FALSE, "Reset Bias"=TRUE}, "Backward sweep"=TRUE, "Number of points"=512, "Channels"=["Current (A)", "LI Demod 1 X (A)", "LI Demod 1 Y (A)", "LI Demod 2 X (A)", "LI Demod 2 Y (A)"], "Parameters"=["X (m)", "Y (m)", "Z (m)", "Z offset (m)", "Settling time (s)", "Integration time (s)", "Z-Ctrl hold", "Final Z (m)"], "Fixed parameters"=["Sweep Start", "Sweep End"], "Multiple sweeps configuration"={"Number of Sweeps"=1, "Save all"=FALSE}, "Initialization"={"Z averaging time (s)"=0.001, "Z offset (m)"=0.0, "Initial settling time (s)"=0.2}, "Sweep Timing"={"Max. slew rate (V/s)"=inf, "Settling time (s)"=0.0082, "Integration time (s)"=0.041}, "End of Sweep"={"End settling time (s)"=5e-05, "Z control time (s)"=5e-05}, "Start value (V)"=-3.0, "End value (V)"=2.0, "Channels 2"=[0, 20, 21, 22, 23], "Name"="Quick_Lockin"}]
  in  "Save As":string
  in  "Zspecparam.txt location":path=path "D:/Scripts/STSparam - Copy (2).txt"
  in  "Save As 2":string
  in  "STSparam.txt location":path=path "D:/Scripts/STSparam.txt"
  in  "Update STS/Zspec Param List":bool
  in  "START EXPERIMENT":bool
  in  "stop":bool
  in  "Duplicate Page 1":bool
  in  "No. of Exp":dbl=2.0 caption="No. of Experiments \n(If more than 5, edit VI)" step=1.0
  in  "Tab Control":T3(tab)=enum."Page 2"
  in  "Experiment 1":T4={"Drift Correction Settings"={"Drift Correction every"=4, "Drift correction Pixels"=128, "Channel index (0-23)"=0, "MaxImagesBack"=2, "Threshold"=2, "Increment"=1, "max applied Drift Correction"=40, "Correct Drift"=TRUE, "Correlate"=0, "Correct z drift"=FALSE, "zdrift \nDuration (s)"=0.0}, "Spectroscopy Setting"={"Imaging Current"=5e-11, "ref Current"=5e-12, "tip Speed (m/s)"=2e-09, "Imaging Bias"=-2.4, "ref Bias"=-0.02, "preSTS delay [ms]"=500, "STS z offset"=2e-10, "during Spec Bias (V)"=-0.02, "trigger1 < Hz"=0.0, "trigger 2 >Hz"=0.0, "autoStop"=FALSE, "Spectroscopy"=0, "PLL ON/OFF"=FALSE, "readjust setpoint every "=1, "z Reference"=TRUE, "Lock In"=FALSE}, "Misc"={"File name"="DCA_Zdependence_STS_Neg_Bias_Mol5_1_zOffset=200pm", "Email when finished"="Dhaneesh.Gopalakrishnan@monash.edu"}, "Grid Settings"={"type"=0, "type order"=0, "X pixel"=6, "Y pixel"=1, "Grid_Parms"={"center X (m)"=0.0, "center Y (m)"=0.0, "width (m)"=0.0, "height (m)"=0.0, "angle (deg)"=0.0}}, "STS Param List #1 "=4, "ZSpec Param List #1  "=0, "Repeat Experiment"={"Repeat"=TRUE, "Repeat Parameter"=2, "Values List #1"=14}} {"Repeat Experiment"."Repeat Parameter" items=["ref Current", "ref Bias", "STS z offset", "during Spec Bias (V)"]; "STS Param List #1" items=["numerical_DCA_-20mV->-3V", "numerical_DCA_-20mV->0.7V", "numerical_DCA_-20mV->-0.7V_30sweeps", "numerical_DCA_-20mV->-0.7V_50_sweeps", "numerical_DCA_-20mV->-3V_70sweeps", "numerical_DCA_-20mV->3V_100_sweeps", "KPFM_MgPc", "KPFM_MgPc2", "KPFM_MgPc_marina", "numerical_-1V->2V", "numerical_-20mV->20mV", "DCA_numerical_-0.2V->0.8V", "numerical_-2V->2.2V", "DCA_numerical2_-0.2V->0.8V", "lockin_-20mV->20mV", "lockin_-25mV->25mV", "test", "lockin_highRes_20mV_-20mV", "lockin_slow", "Lock_in_DCA_1.5V->-50mV", "Long_MgPc_lockin_-1->1V", "MgPc_long_lockin", "lockin_slow_-1_2", "MgPc_long_lockin2", "Quick_Lockin"]; "Grid Settings"."type order" items=["Grid", "Random", "Adam7"]; "Grid Settings"."type" items=["Line", "Grid", "Cloud"]; "Spectroscopy Setting"."Spectroscopy" items=["Bias", "zSpec"]; "Spectroscopy Setting"."trigger 2 >Hz" format="%#_6p"; "Spectroscopy Setting"."trigger1 < Hz" format="%#_6p"; "Spectroscopy Setting"."during Spec Bias (V)" format="%#_5p"; "Spectroscopy Setting"."STS z offset" format="%#_6p"; "Spectroscopy Setting"."ref Bias" format="%#_6p"; "Spectroscopy Setting"."Imaging Bias" format="%#_6p"; "Spectroscopy Setting"."tip Speed (m/s)" format="%.2p"; "Spectroscopy Setting"."ref Current" format="%#_6p"; "Spectroscopy Setting"."Imaging Current" format="%#_6p"; "Drift Correction Settings"."Correlate" items=["first Frame", "successive Frames"]; "Drift Correction Settings"."max applied Drift Correction" min=1 max=100 step=1 format="%.0p"; "Drift Correction Settings"."Threshold" min=1 step=1; "Drift Correction Settings"."Channel index (0-23)" items=["Current"=0, "Z (m)"=14]}
  in  "Experiment 2":T5={"Drift Correction Settings"={"Drift Correction every"=1, "Drift correction Pixels"=128, "Channel index (0-23)"=0, "MaxImagesBack"=2, "Threshold"=2, "Increment"=1, "max applied Drift Correction"=40, "Correct Drift"=TRUE, "Correlate"=0, "Correct z drift"=FALSE, "zdrift \nDuration (s)"=0.0}, "Spectroscopy Setting"={"Imaging Current"=5e-11, "ref Current"=5e-12, "tip Speed (m/s)"=2e-09, "Imaging Bias"=-2.4, "ref Bias"=-0.02, "preSTS delay [ms]"=500, "STS z offset"=0.0, "during Spec Bias (V)"=-0.02, "trigger1 < Hz"=0.0, "trigger 2 >Hz"=0.0, "autoStop"=FALSE, "Spectroscopy"=0, "PLL ON/OFF"=FALSE, "readjust setpoint every "=1, "z Reference"=TRUE, "Lock In"=FALSE}, "Misc"={"File name"="DCA_Zdependence_STS_Neg_Bias_Mol5_1", "Email when finished"="Dhaneesh.Gopalakrishnan@monash.edu"}, "Grid Settings"={"type"=0, "type order"=0, "X pixel"=6, "Y pixel"=1, "Grid_Parms"={"center X (m)"=0.0, "center Y (m)"=0.0, "width (m)"=0.0, "height (m)"=0.0, "angle (deg)"=0.0}}, "STS Param List #2 "=0, "ZSpec Param List  #2 "=0, "Repeat Experiment"={"Repeat"=TRUE, "Repeat Parameter"=2, "Values List #2"=7}} {"Repeat Experiment"."Repeat Parameter" items=["ref Current", "ref Bias", "STS z offset", "during Spec Bias (V)"]; "STS Param List #2" items=["numerical_DCA_-20mV->-3V", "numerical_DCA_-20mV->0.7V", "numerical_DCA_-20mV->-0.7V_30sweeps", "numerical_DCA_-20mV->-0.7V_50_sweeps", "numerical_DCA_-20mV->-3V_70sweeps", "numerical_DCA_-20mV->3V_100_sweeps", "KPFM_MgPc", "KPFM_MgPc2", "KPFM_MgPc_marina", "numerical_-1V->2V", "numerical_-20mV->20mV", "DCA_numerical_-0.2V->0.8V", "numerical_-2V->2.2V", "DCA_numerical2_-0.2V->0.8V", "lockin_-20mV->20mV", "lockin_-25mV->25mV", "test", "lockin_highRes_20mV_-20mV", "lockin_slow", "Lock_in_DCA_1.5V->-50mV", "Long_MgPc_lockin_-1->1V", "MgPc_long_lockin", "lockin_slow_-1_2", "MgPc_long_lockin2", "Quick_Lockin"]; "Grid Settings"."type order" items=["Grid", "Random", "Adam7"]; "Grid Settings"."type" items=["Line", "Grid", "Cloud"]; "Spectroscopy Setting"."Spectroscopy" items=["Bias", "zSpec"]; "Spectroscopy Setting"."trigger 2 >Hz" format="%#_6p"; "Spectroscopy Setting"."trigger1 < Hz" format="%#_6p"; "Spectroscopy Setting"."during Spec Bias (V)" format="%#_5p"; "Spectroscopy Setting"."STS z offset" format="%#_6p"; "Spectroscopy Setting"."ref Bias" format="%#_6p"; "Spectroscopy Setting"."Imaging Bias" format="%#_6p"; "Spectroscopy Setting"."tip Speed (m/s)" format="%.2p"; "Spectroscopy Setting"."ref Current" format="%#_6p"; "Spectroscopy Setting"."Imaging Current" format="%#_6p"; "Drift Correction Settings"."Correlate" items=["first Frame", "successive Frames"]; "Drift Correction Settings"."max applied Drift Correction" min=1 max=100 step=1 format="%.0p"; "Drift Correction Settings"."Threshold" min=1 step=1; "Drift Correction Settings"."Channel index (0-23)" items=["Current"=0, "Z (m)"=14]}
  in  "Experiment 3":T6={"Drift Correction Settings"={"Drift Correction every"=6, "Drift correction Pixels"=128, "Channel index (0-23)"=0, "MaxImagesBack"=2, "Threshold"=2, "Increment"=1, "max applied Drift Correction"=40, "Correct Drift"=TRUE, "Correlate"=0, "Correct z drift"=FALSE, "zdrift \nDuration (s)"=0.0}, "Spectroscopy Setting"={"Imaging Current"=5e-11, "ref Current"=5e-12, "tip Speed (m/s)"=2e-09, "Imaging Bias"=-2.4, "ref Bias"=-0.02, "preSTS delay [ms]"=500, "STS z offset"=4e-10, "during Spec Bias (V)"=-0.02, "trigger1 < Hz"=0.0, "trigger 2 >Hz"=0.0, "autoStop"=FALSE, "Spectroscopy"=0, "PLL ON/OFF"=FALSE, "readjust setpoint every "=1, "z Reference"=TRUE, "Lock In"=FALSE}, "Misc"={"File name"="DCA_Zdependence_STS_Neg_Bias_Mol5_1", "Email when finished"="Dhaneesh.Gopalakrishnan@monash.edu"}, "Grid Settings"={"type"=0, "type order"=0, "X pixel"=6, "Y pixel"=1, "Grid_Parms"={"center X (m)"=0.0, "center Y (m)"=0.0, "width (m)"=0.0, "height (m)"=0.0, "angle (deg)"=0.0}}, "STS Param List #3 "=4, "ZSpec Param List #3 "=0, "Repeat Experiment"={"Repeat"=TRUE, "Repeat Parameter"=2, "Values List #3"=7}} {"Repeat Experiment"."Repeat Parameter" items=["ref Current", "ref Bias", "STS z offset", "during Spec Bias (V)"]; "STS Param List #3" items=["numerical_DCA_-20mV->-3V", "numerical_DCA_-20mV->0.7V", "numerical_DCA_-20mV->-0.7V_30sweeps", "numerical_DCA_-20mV->-0.7V_50_sweeps", "numerical_DCA_-20mV->-3V_70sweeps", "numerical_DCA_-20mV->3V_100_sweeps", "KPFM_MgPc", "KPFM_MgPc2", "KPFM_MgPc_marina", "numerical_-1V->2V", "numerical_-20mV->20mV", "DCA_numerical_-0.2V->0.8V", "numerical_-2V->2.2V", "DCA_numerical2_-0.2V->0.8V", "lockin_-20mV->20mV", "lockin_-25mV->25mV", "test", "lockin_highRes_20mV_-20mV", "lockin_slow", "Lock_in_DCA_1.5V->-50mV", "Long_MgPc_lockin_-1->1V", "MgPc_long_lockin", "lockin_slow_-1_2", "MgPc_long_lockin2", "Quick_Lockin"]; "Grid Settings"."type order" items=["Grid", "Random", "Adam7"]; "Grid Settings"."type" items=["Line", "Grid", "Cloud"]; "Spectroscopy Setting"."Spectroscopy" items=["Bias", "zSpec"]; "Spectroscopy Setting"."trigger 2 >Hz" format="%#_6p"; "Spectroscopy Setting"."trigger1 < Hz" format="%#_6p"; "Spectroscopy Setting"."during Spec Bias (V)" format="%#_5p"; "Spectroscopy Setting"."STS z offset" format="%#_6p"; "Spectroscopy Setting"."ref Bias" format="%#_6p"; "Spectroscopy Setting"."Imaging Bias" format="%#_6p"; "Spectroscopy Setting"."tip Speed (m/s)" format="%.2p"; "Spectroscopy Setting"."ref Current" format="%#_6p"; "Spectroscopy Setting"."Imaging Current" format="%#_6p"; "Drift Correction Settings"."Correlate" items=["first Frame", "successive Frames"]; "Drift Correction Settings"."max applied Drift Correction" min=1 max=100 step=1 format="%.0p"; "Drift Correction Settings"."Threshold" min=1 step=1; "Drift Correction Settings"."Channel index (0-23)" items=["Current"=0, "Z (m)"=14]}
  in  "Experiment 4":T7={"Drift Correction Settings"={"Drift Correction every"=1, "Drift correction Pixels"=128, "Channel index (0-23)"=0, "MaxImagesBack"=2, "Threshold"=2, "Increment"=1, "max applied Drift Correction"=40, "Correct Drift"=TRUE, "Correlate"=0, "Correct z drift"=FALSE, "zdrift \nDuration (s)"=0.0}, "Spectroscopy Setting"={"Imaging Current"=5e-11, "ref Current"=5e-12, "tip Speed (m/s)"=1e-08, "Imaging Bias"=-2.4, "ref Bias"=-0.02, "preSTS delay [ms]"=500, "STS z offset"=0.0, "during Spec Bias (V)"=-0.02, "trigger1 < Hz"=0.0, "trigger 2 >Hz"=0.0, "autoStop"=FALSE, "Spectroscopy"=0, "PLL ON/OFF"=FALSE, "readjust setpoint every "=1, "z Reference"=TRUE, "Lock In"=FALSE}, "Misc"={"File name"="DCA_Zdependence_STS_Neg_Bias_Mol5_1", "Email when finished"="Dhaneesh.Gopalakrishnan@monash.edu"}, "Grid Settings"={"type"=0, "type order"=0, "X pixel"=6, "Y pixel"=1, "Grid_Parms"={"center X (m)"=0.0, "center Y (m)"=0.0, "width (m)"=0.0, "height (m)"=0.0, "angle (deg)"=0.0}}, "STS Param List #4 "=0, "ZSpec Param List  #4"=0, "Repeat Experiment"={"Repeat"=TRUE, "Repeat Parameter"=2, "Values List #4"=7}} {"Repeat Experiment"."Repeat Parameter" items=["ref Current", "ref Bias", "STS z offset", "during Spec Bias (V)"]; "STS Param List #4" items=["numerical_DCA_-20mV->-3V", "numerical_DCA_-20mV->0.7V", "numerical_DCA_-20mV->-0.7V_30sweeps", "numerical_DCA_-20mV->-0.7V_50_sweeps", "numerical_DCA_-20mV->-3V_70sweeps", "numerical_DCA_-20mV->3V_100_sweeps", "KPFM_MgPc", "KPFM_MgPc2", "KPFM_MgPc_marina", "numerical_-1V->2V", "numerical_-20mV->20mV", "DCA_numerical_-0.2V->0.8V", "numerical_-2V->2.2V", "DCA_numerical2_-0.2V->0.8V", "lockin_-20mV->20mV", "lockin_-25mV->25mV", "test", "lockin_highRes_20mV_-20mV", "lockin_slow", "Lock_in_DCA_1.5V->-50mV", "Long_MgPc_lockin_-1->1V", "MgPc_long_lockin", "lockin_slow_-1_2", "MgPc_long_lockin2", "Quick_Lockin"]; "Grid Settings"."type order" items=["Grid", "Random", "Adam7"]; "Grid Settings"."type" items=["Line", "Grid", "Cloud"]; "Spectroscopy Setting"."Spectroscopy" items=["Bias", "zSpec"]; "Spectroscopy Setting"."trigger 2 >Hz" format="%#_6p"; "Spectroscopy Setting"."trigger1 < Hz" format="%#_6p"; "Spectroscopy Setting"."during Spec Bias (V)" format="%#_5p"; "Spectroscopy Setting"."STS z offset" format="%#_6p"; "Spectroscopy Setting"."ref Bias" format="%#_6p"; "Spectroscopy Setting"."Imaging Bias" format="%#_6p"; "Spectroscopy Setting"."tip Speed (m/s)" format="%.2p"; "Spectroscopy Setting"."ref Current" format="%#_6p"; "Spectroscopy Setting"."Imaging Current" format="%#_6p"; "Drift Correction Settings"."Correlate" items=["first Frame", "successive Frames"]; "Drift Correction Settings"."max applied Drift Correction" min=1 max=100 step=1 format="%.0p"; "Drift Correction Settings"."Threshold" min=1 step=1; "Drift Correction Settings"."Channel index (0-23)" items=["Current"=0, "Z (m)"=14]}
  in  "Experiment 5":T8={"Drift Correction Settings"={"Drift Correction every"=1, "Drift correction Pixels"=256, "Channel index (0-23)"=0, "MaxImagesBack"=2, "Threshold"=2, "Increment"=1, "max applied Drift Correction"=40, "Correct Drift"=TRUE, "Correlate"=0, "Correct z drift"=FALSE, "zdrift \nDuration (s)"=0.0}, "Spectroscopy Setting"={"Imaging Current"=5e-11, "ref Current"=5e-12, "tip Speed (m/s)"=1e-08, "Imaging Bias"=-2.4, "ref Bias"=-0.02, "preSTS delay [ms]"=500, "STS z offset"=0.0, "during Spec Bias (V)"=-0.02, "trigger1 < Hz"=0.0, "trigger 2 >Hz"=0.0, "autoStop"=FALSE, "Spectroscopy"=0, "PLL ON/OFF"=FALSE, "readjust setpoint every "=1, "z Reference"=TRUE, "Lock In"=FALSE}, "Misc"={"File name"="DCA_Zdependence_STS_Pos_Bias_Mol9_46", "Email when finished"="Dhaneesh.Gopalakrishnan@monash.edu"}, "Grid Settings"={"type"=0, "type order"=0, "X pixel"=27, "Y pixel"=1, "Grid_Parms"={"center X (m)"=0.0, "center Y (m)"=0.0, "width (m)"=0.0, "height (m)"=0.0, "angle (deg)"=0.0}}, "STS Param List #5 "=0, "ZSpec Param List #5  "=0, "Repeat Experiment"={"Repeat"=TRUE, "Repeat Parameter"=2, "Values List #5"=7}} {"Repeat Experiment"."Repeat Parameter" items=["ref Current", "ref Bias", "STS z offset", "during Spec Bias (V)"]; "STS Param List #5" items=["numerical_DCA_-20mV->-3V", "numerical_DCA_-20mV->0.7V", "numerical_DCA_-20mV->-0.7V_30sweeps", "numerical_DCA_-20mV->-0.7V_50_sweeps", "numerical_DCA_-20mV->-3V_70sweeps", "numerical_DCA_-20mV->3V_100_sweeps", "KPFM_MgPc", "KPFM_MgPc2", "KPFM_MgPc_marina", "numerical_-1V->2V", "numerical_-20mV->20mV", "DCA_numerical_-0.2V->0.8V", "numerical_-2V->2.2V", "DCA_numerical2_-0.2V->0.8V", "lockin_-20mV->20mV", "lockin_-25mV->25mV", "test", "lockin_highRes_20mV_-20mV", "lockin_slow", "Lock_in_DCA_1.5V->-50mV", "Long_MgPc_lockin_-1->1V", "MgPc_long_lockin", "lockin_slow_-1_2", "MgPc_long_lockin2", "Quick_Lockin"]; "Grid Settings"."type order" items=["Grid", "Random", "Adam7"]; "Grid Settings"."type" items=["Line", "Grid", "Cloud"]; "Spectroscopy Setting"."Spectroscopy" items=["Bias", "zSpec"]; "Spectroscopy Setting"."trigger 2 >Hz" format="%#_6p"; "Spectroscopy Setting"."trigger1 < Hz" format="%#_6p"; "Spectroscopy Setting"."during Spec Bias (V)" format="%#_5p"; "Spectroscopy Setting"."STS z offset" format="%#_6p"; "Spectroscopy Setting"."ref Bias" format="%#_6p"; "Spectroscopy Setting"."Imaging Bias" format="%#_6p"; "Spectroscopy Setting"."tip Speed (m/s)" format="%.2p"; "Spectroscopy Setting"."ref Current" format="%#_6p"; "Spectroscopy Setting"."Imaging Current" format="%#_6p"; "Drift Correction Settings"."Correlate" items=["first Frame", "successive Frames"]; "Drift Correction Settings"."max applied Drift Correction" min=1 max=100 step=1 format="%.0p"; "Drift Correction Settings"."Threshold" min=1 step=1; "Drift Correction Settings"."Channel index (0-23)" items=["Current"=0, "Z (m)"=14]}
  # "z Spectroscopy"
  # "GRID points"
  # "Increase this if no Drift was detected for \na certain number of images"
  # "% of image size"
  # "Only first frame works"
  # "z Spectroscopy"
  # "GRID points"
  # "Increase this if no Drift was detected for \na certain number of images"
  # "% of image size"
  # "Only first frame works"
  # "z Spectroscopy"
  # "GRID points"
  # "Increase this if no Drift was detected for \na certain number of images"
  # "% of image size"
  # "Only first frame works"
  # "z Spectroscopy"
  # "GRID points"
  # "Increase this if no Drift was detected for \na certain number of images"
  # "% of image size"
  # "Only first frame works"
  # "z Spectroscopy"
  # "GRID points"
  # "Increase this if no Drift was detected for \na certain number of images"
  # "% of image size"
  # "Only first frame works"
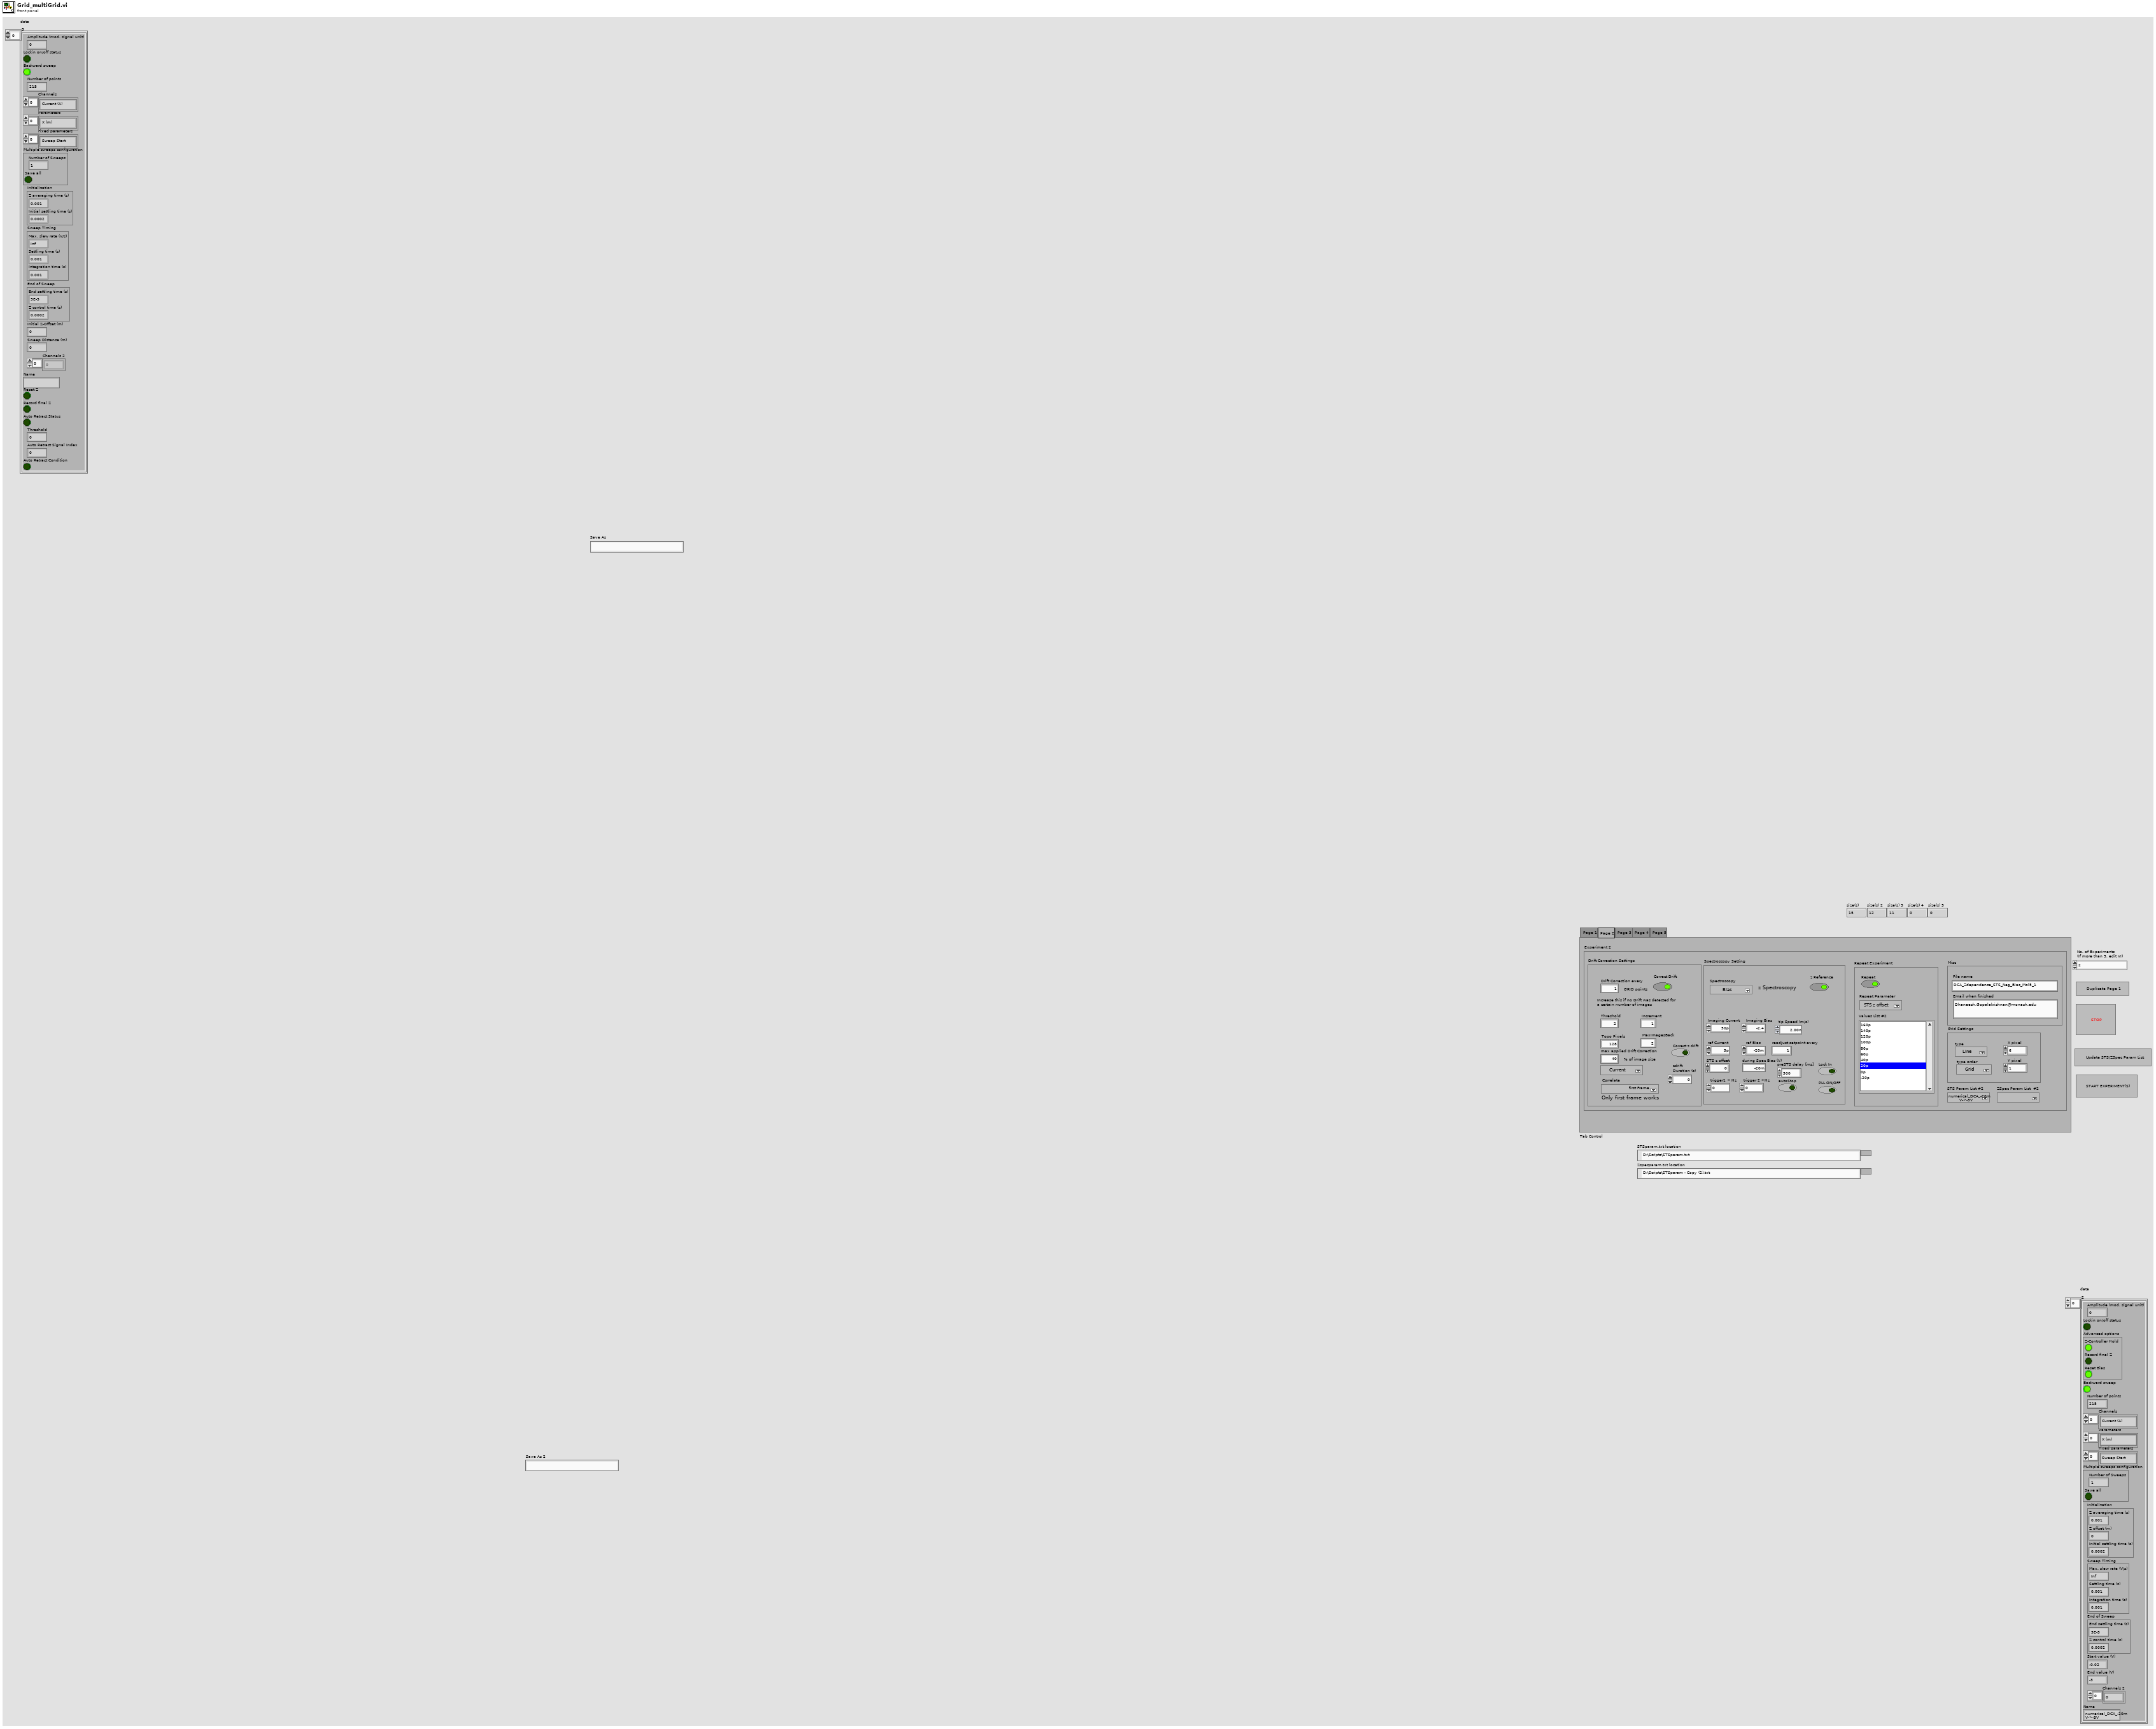
[diagram p1: front panel]
types:
  T1 = cluster{"Amplitude (mod. signal unit)":sgl, "Lockin on/off status":bool, "Backward sweep":bool, "Number of points":i32, "Channels":string[], "Parameters":string[], "Fixed parameters":string[], "Multiple sweeps configuration":cluster{"Number of Sweeps":i32, "Save all":bool}, "Initialization":cluster{"Z averaging time (s)":sgl, "Initial settling time (s)":sgl}, "Sweep Timing":cluster{"Max. slew rate (V/s)":sgl, "Settling time (s)":sgl, "Integration time (s)":sgl}, "End of Sweep":cluster{"End settling time (s)":sgl, "Z control time (s)":sgl}, "Initial Z-Offset (m)":sgl, "Sweep Distance (m)":sgl, "Channels 2":i32[], "Name":string, "Reset Z":bool, "Record final Z":bool, "Auto Retract Status":bool, "Threshold":sgl, "Auto Retract Signal Index":i32, "Auto Retract Condition":bool}[]
  T2 = cluster{"Amplitude (mod. signal unit)":sgl, "Lockin on/off status":bool, "Advanced options":cluster{"Z-Controller Hold":bool, "Record final Z":bool, "Reset Bias":bool}, "Backward sweep":bool, "Number of points":i32, "Channels":string[], "Parameters":string[], "Fixed parameters":string[], "Multiple sweeps configuration":cluster{"Number of Sweeps":i32, "Save all":bool}, "Initialization":cluster{"Z averaging time (s)":sgl, "Z offset (m)":sgl, "Initial settling time (s)":sgl}, "Sweep Timing":cluster{"Max. slew rate (V/s)":sgl, "Settling time (s)":sgl, "Integration time (s)":sgl}, "End of Sweep":cluster{"End settling time (s)":sgl, "Z control time (s)":sgl}, "Start value (V)":sgl, "End value (V)":sgl, "Channels 2":i32[], "Name":string}[]
  T3 = enum32{"Page 1", "Page 2", "Page 3", "Page 4", "Page 5"}
  T4 = cluster{"Drift Correction Settings":cluster{"Drift Correction every":i32, "Drift correction Pixels":i32, "Channel index (0-23)":u8, "MaxImagesBack":i32, "Threshold":i32, "Increment":i32, "max applied Drift Correction":i32, "Correct Drift":bool, "Correlate":u16, "Correct z drift":bool, "zdrift \nDuration (s)":dbl}, "Spectroscopy Setting":cluster{"Imaging Current":dbl, "ref Current":dbl, "tip Speed (m/s)":sgl, "Imaging Bias":dbl, "ref Bias":dbl, "preSTS delay [ms]":u32, "STS z offset":dbl, "during Spec Bias (V)":sgl, "trigger1 < Hz":sgl, "trigger 2 >Hz":sgl, "autoStop":bool, "Spectroscopy":u16, "PLL ON/OFF":bool, "readjust setpoint every ":i32, "z Reference":bool, "Lock In":bool}, "Misc":cluster{"File name":string, "Email when finished":string}, "Grid Settings":cluster{"type":u16, "type order":u16, "X pixel":i32, "Y pixel":i32, "Grid_Parms":cluster{"center X (m)":sgl, "center Y (m)":sgl, "width (m)":sgl, "height (m)":sgl, "angle (deg)":sgl}}, "STS Param List #1 ":u16, "ZSpec Param List #1  ":u16, "Repeat Experiment":cluster{"Repeat":bool, "Repeat Parameter":u16, "Values List #1":i32}}
  T5 = cluster{"Drift Correction Settings":cluster{"Drift Correction every":i32, "Drift correction Pixels":i32, "Channel index (0-23)":u8, "MaxImagesBack":i32, "Threshold":i32, "Increment":i32, "max applied Drift Correction":i32, "Correct Drift":bool, "Correlate":u16, "Correct z drift":bool, "zdrift \nDuration (s)":dbl}, "Spectroscopy Setting":cluster{"Imaging Current":dbl, "ref Current":dbl, "tip Speed (m/s)":sgl, "Imaging Bias":dbl, "ref Bias":dbl, "preSTS delay [ms]":u32, "STS z offset":dbl, "during Spec Bias (V)":sgl, "trigger1 < Hz":sgl, "trigger 2 >Hz":sgl, "autoStop":bool, "Spectroscopy":u16, "PLL ON/OFF":bool, "readjust setpoint every ":i32, "z Reference":bool, "Lock In":bool}, "Misc":cluster{"File name":string, "Email when finished":string}, "Grid Settings":cluster{"type":u16, "type order":u16, "X pixel":i32, "Y pixel":i32, "Grid_Parms":cluster{"center X (m)":sgl, "center Y (m)":sgl, "width (m)":sgl, "height (m)":sgl, "angle (deg)":sgl}}, "STS Param List #2 ":u16, "ZSpec Param List  #2 ":u16, "Repeat Experiment":cluster{"Repeat":bool, "Repeat Parameter":u16, "Values List #2":i32}}
  T6 = cluster{"Drift Correction Settings":cluster{"Drift Correction every":i32, "Drift correction Pixels":i32, "Channel index (0-23)":u8, "MaxImagesBack":i32, "Threshold":i32, "Increment":i32, "max applied Drift Correction":i32, "Correct Drift":bool, "Correlate":u16, "Correct z drift":bool, "zdrift \nDuration (s)":dbl}, "Spectroscopy Setting":cluster{"Imaging Current":dbl, "ref Current":dbl, "tip Speed (m/s)":sgl, "Imaging Bias":dbl, "ref Bias":dbl, "preSTS delay [ms]":u32, "STS z offset":dbl, "during Spec Bias (V)":sgl, "trigger1 < Hz":sgl, "trigger 2 >Hz":sgl, "autoStop":bool, "Spectroscopy":u16, "PLL ON/OFF":bool, "readjust setpoint every ":i32, "z Reference":bool, "Lock In":bool}, "Misc":cluster{"File name":string, "Email when finished":string}, "Grid Settings":cluster{"type":u16, "type order":u16, "X pixel":i32, "Y pixel":i32, "Grid_Parms":cluster{"center X (m)":sgl, "center Y (m)":sgl, "width (m)":sgl, "height (m)":sgl, "angle (deg)":sgl}}, "STS Param List #3 ":u16, "ZSpec Param List #3 ":u16, "Repeat Experiment":cluster{"Repeat":bool, "Repeat Parameter":u16, "Values List #3":i32}}
  T7 = cluster{"Drift Correction Settings":cluster{"Drift Correction every":i32, "Drift correction Pixels":i32, "Channel index (0-23)":u8, "MaxImagesBack":i32, "Threshold":i32, "Increment":i32, "max applied Drift Correction":i32, "Correct Drift":bool, "Correlate":u16, "Correct z drift":bool, "zdrift \nDuration (s)":dbl}, "Spectroscopy Setting":cluster{"Imaging Current":dbl, "ref Current":dbl, "tip Speed (m/s)":sgl, "Imaging Bias":dbl, "ref Bias":dbl, "preSTS delay [ms]":u32, "STS z offset":dbl, "during Spec Bias (V)":sgl, "trigger1 < Hz":sgl, "trigger 2 >Hz":sgl, "autoStop":bool, "Spectroscopy":u16, "PLL ON/OFF":bool, "readjust setpoint every ":i32, "z Reference":bool, "Lock In":bool}, "Misc":cluster{"File name":string, "Email when finished":string}, "Grid Settings":cluster{"type":u16, "type order":u16, "X pixel":i32, "Y pixel":i32, "Grid_Parms":cluster{"center X (m)":sgl, "center Y (m)":sgl, "width (m)":sgl, "height (m)":sgl, "angle (deg)":sgl}}, "STS Param List #4 ":u16, "ZSpec Param List  #4":u16, "Repeat Experiment":cluster{"Repeat":bool, "Repeat Parameter":u16, "Values List #4":i32}}
  T8 = cluster{"Drift Correction Settings":cluster{"Drift Correction every":i32, "Drift correction Pixels":i32, "Channel index (0-23)":u8, "MaxImagesBack":i32, "Threshold":i32, "Increment":i32, "max applied Drift Correction":i32, "Correct Drift":bool, "Correlate":u16, "Correct z drift":bool, "zdrift \nDuration (s)":dbl}, "Spectroscopy Setting":cluster{"Imaging Current":dbl, "ref Current":dbl, "tip Speed (m/s)":sgl, "Imaging Bias":dbl, "ref Bias":dbl, "preSTS delay [ms]":u32, "STS z offset":dbl, "during Spec Bias (V)":sgl, "trigger1 < Hz":sgl, "trigger 2 >Hz":sgl, "autoStop":bool, "Spectroscopy":u16, "PLL ON/OFF":bool, "readjust setpoint every ":i32, "z Reference":bool, "Lock In":bool}, "Misc":cluster{"File name":string, "Email when finished":string}, "Grid Settings":cluster{"type":u16, "type order":u16, "X pixel":i32, "Y pixel":i32, "Grid_Parms":cluster{"center X (m)":sgl, "center Y (m)":sgl, "width (m)":sgl, "height (m)":sgl, "angle (deg)":sgl}}, "STS Param List #5 ":u16, "ZSpec Param List #5  ":u16, "Repeat Experiment":cluster{"Repeat":bool, "Repeat Parameter":u16, "Values List #5":i32}}
  T9 = cluster{"Amplitude (mod. signal unit)":sgl, "Lockin on/off status":bool, "Backward sweep":bool, "Number of points":i32, "Channels":string[], "Parameters":string[], "Fixed parameters":string[], "Multiple sweeps configuration":cluster{"Number of Sweeps":i32, "Save all":bool}, "Initialization":cluster{"Z averaging time (s)":sgl, "Initial settling time (s)":sgl}, "Sweep Timing":cluster{"Max. slew rate (V/s)":sgl, "Settling time (s)":sgl, "Integration time (s)":sgl}, "End of Sweep":cluster{"End settling time (s)":sgl, "Z control time (s)":sgl}, "Initial Z-Offset (m)":sgl, "Sweep Distance (m)":sgl, "Channels 2":i32[], "Name":string, "Reset Z":bool, "Record final Z":bool, "Auto Retract Status":bool, "Threshold":sgl, "Auto Retract Signal Index":i32, "Auto Retract Condition":bool}
  T10 = cluster{"Amplitude (mod. signal unit)":sgl, "Lockin on/off status":bool, "Advanced options":cluster{"Z-Controller Hold":bool, "Record final Z":bool, "Reset Bias":bool}, "Backward sweep":bool, "Number of points":i32, "Channels":string[], "Parameters":string[], "Fixed parameters":string[], "Multiple sweeps configuration":cluster{"Number of Sweeps":i32, "Save all":bool}, "Initialization":cluster{"Z averaging time (s)":sgl, "Z offset (m)":sgl, "Initial settling time (s)":sgl}, "Sweep Timing":cluster{"Max. slew rate (V/s)":sgl, "Settling time (s)":sgl, "Integration time (s)":sgl}, "End of Sweep":cluster{"End settling time (s)":sgl, "Z control time (s)":sgl}, "Start value (V)":sgl, "End value (V)":sgl, "Channels 2":i32[], "Name":string}
  T11 = cluster{"Drift Correction every":i32, "Drift correction Pixels":i32, "Channel index (0-23)":u8, "MaxImagesBack":i32, "Threshold":i32, "Increment":i32, "max applied Drift Correction":i32, "Correct Drift":bool, "Correlate":u16, "Correct z drift":bool, "zdrift \nDuration (s)":dbl}
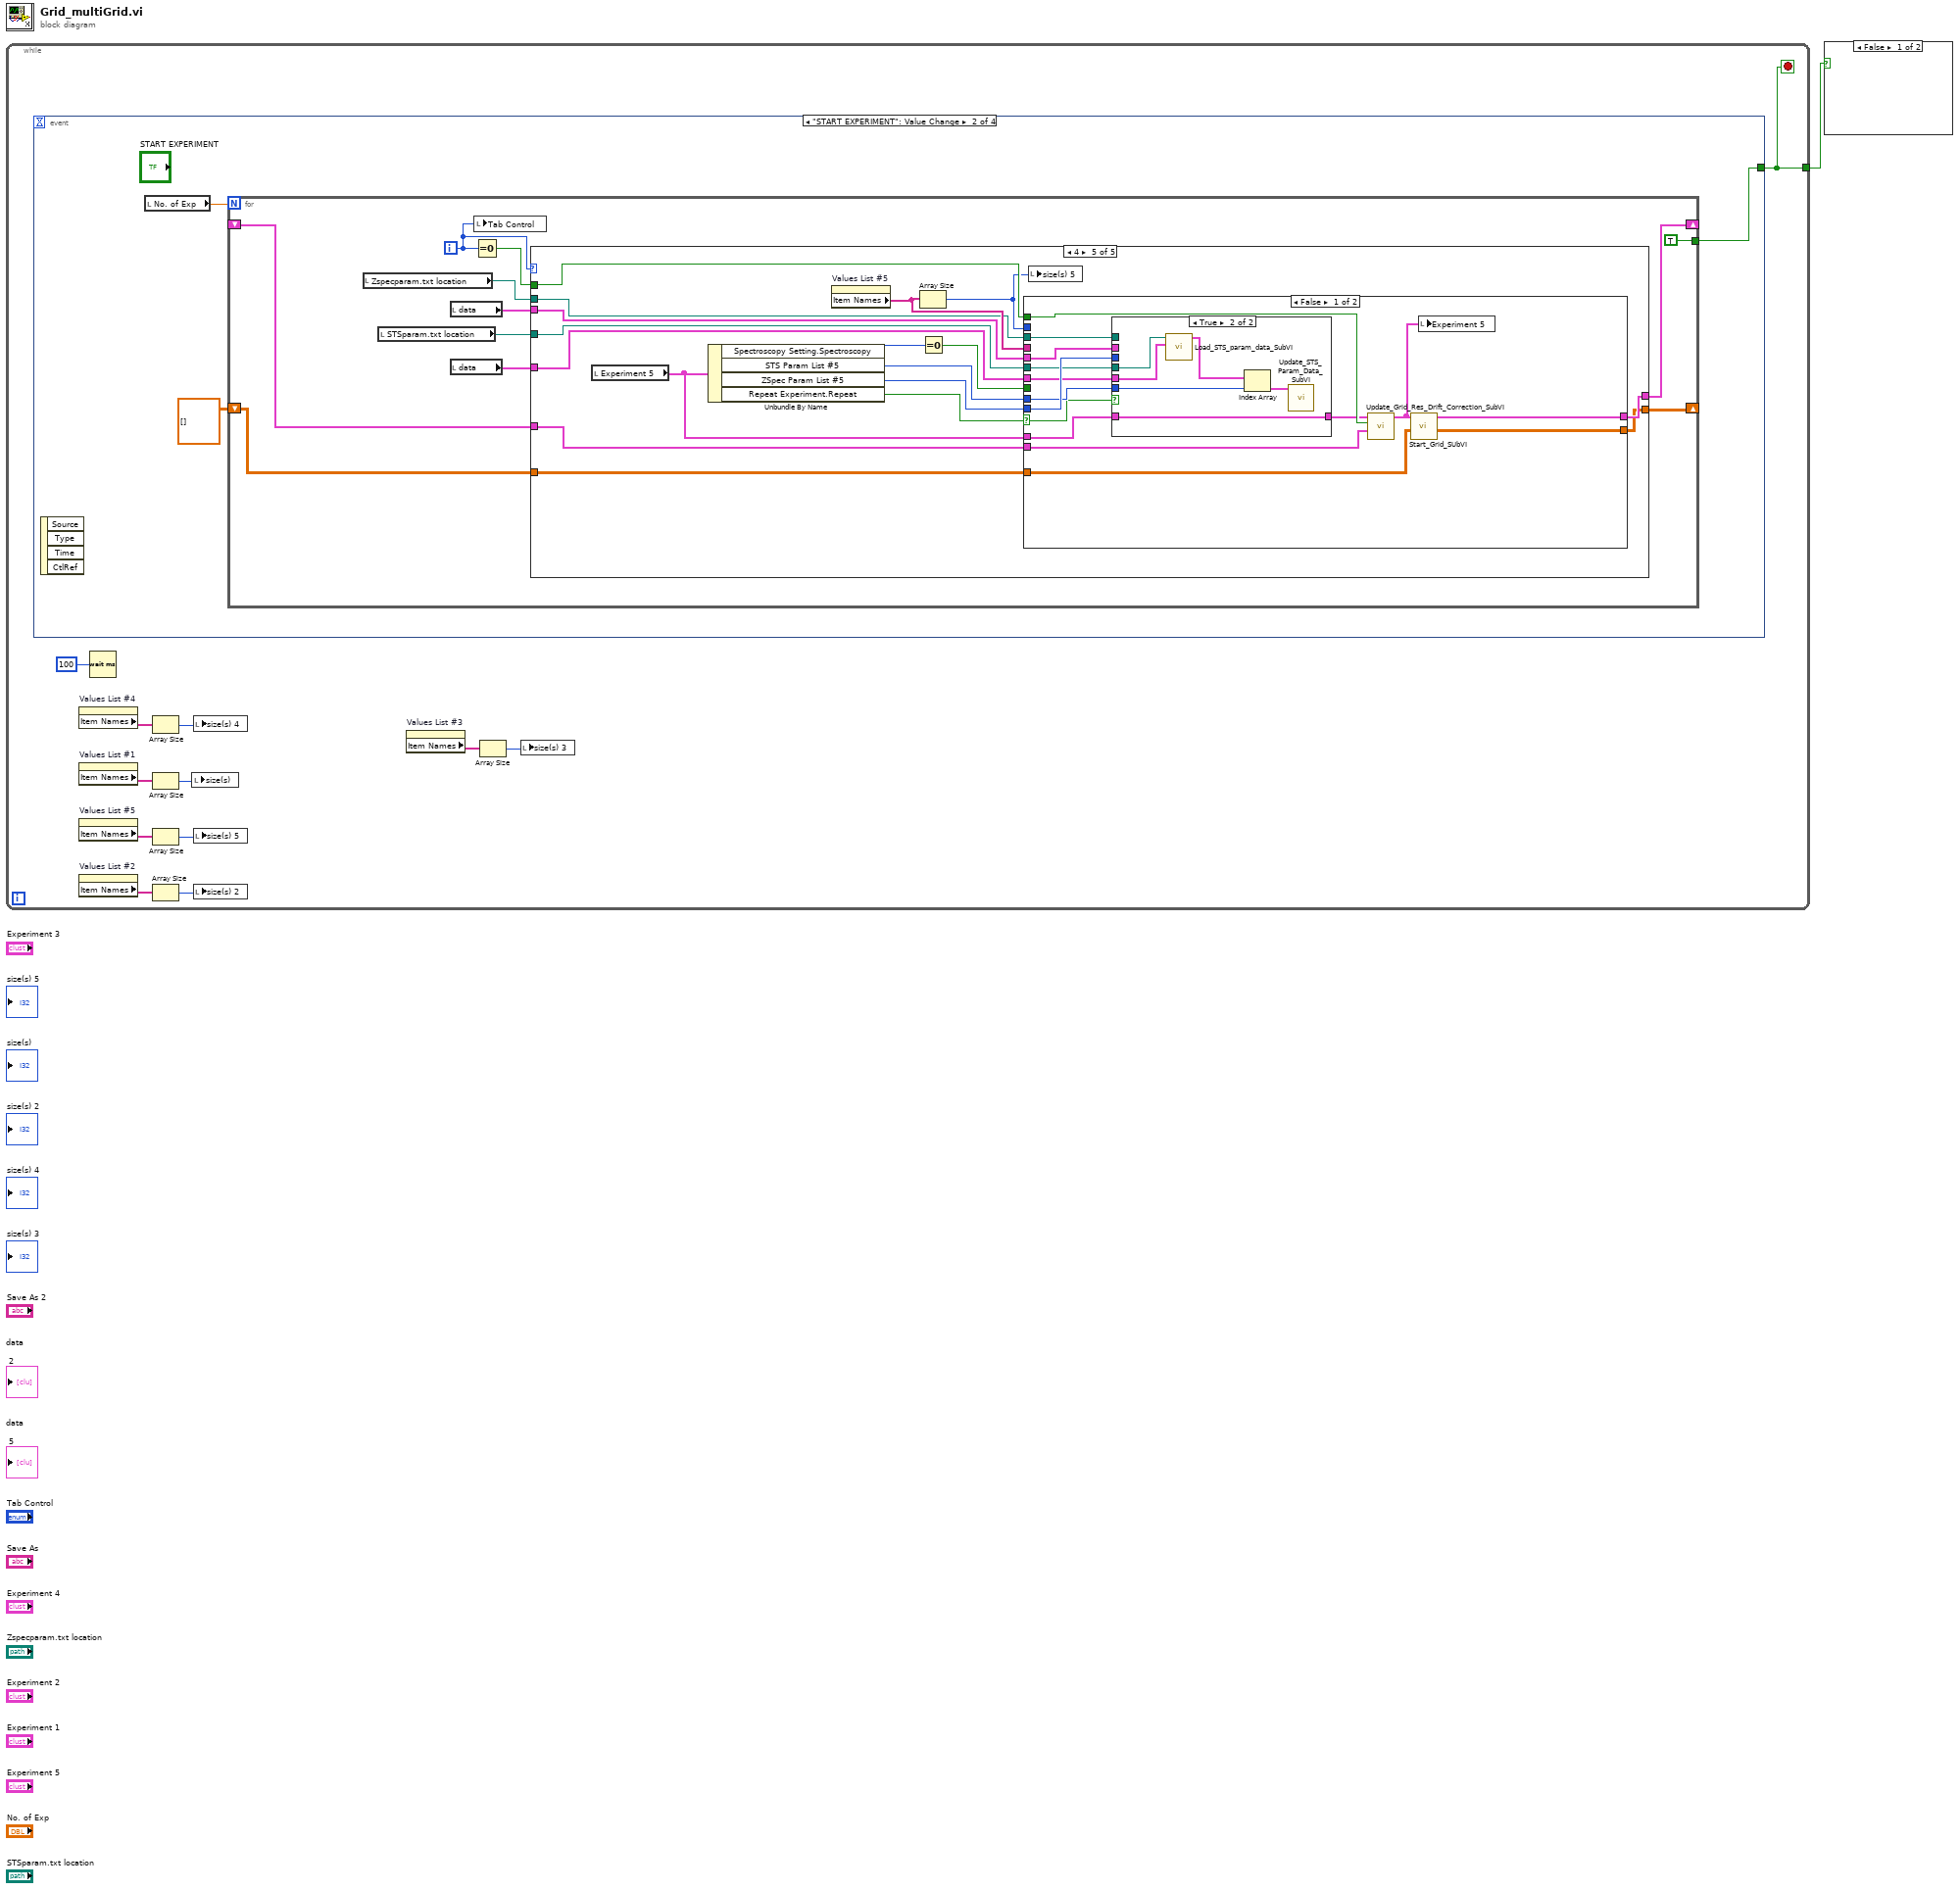
[diagram p0: block diagram]
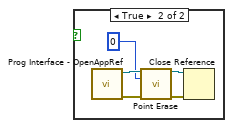
[diagram p2: hidden frame]
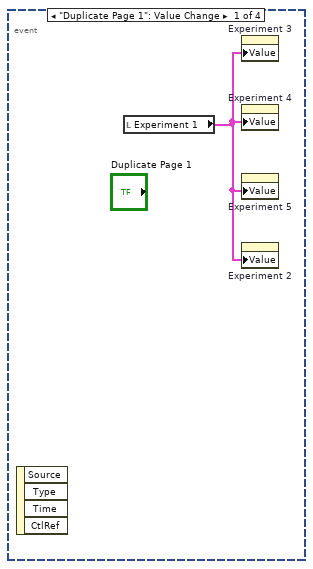
[diagram p3: hidden frame]
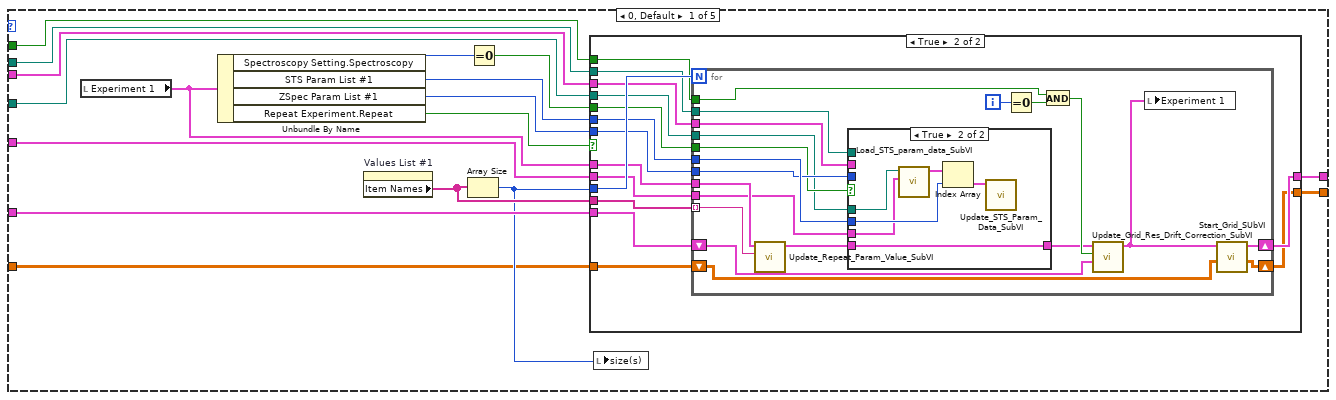
[diagram p4: hidden frame]
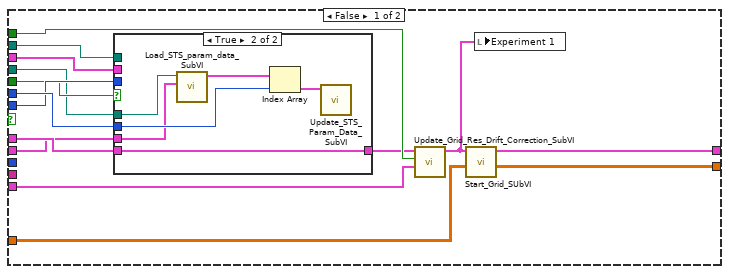
[diagram p5: hidden frame]
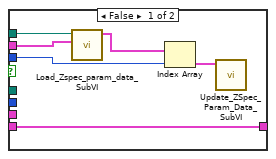
[diagram p6: hidden frame]
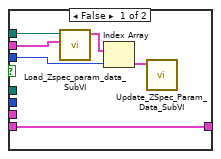
[diagram p7: hidden frame]
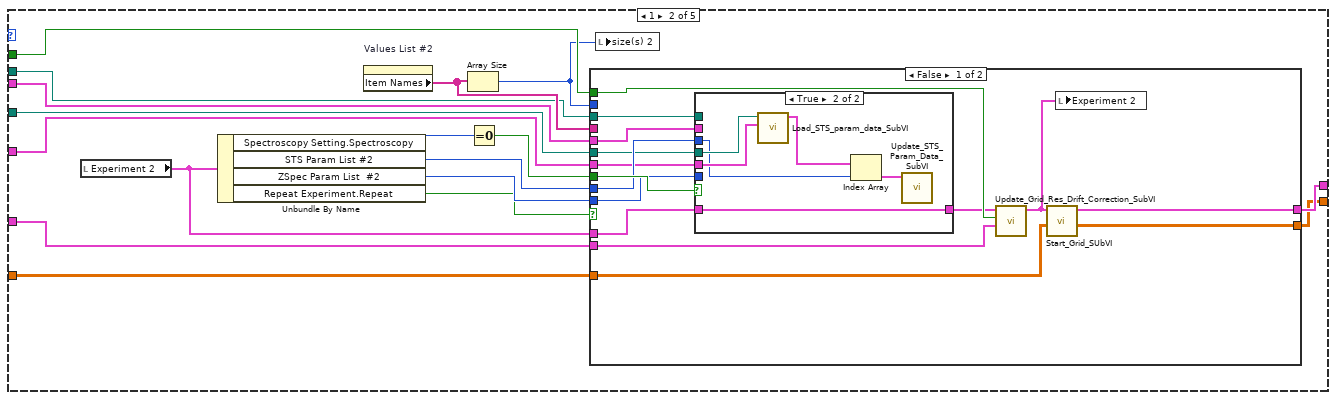
[diagram p8: hidden frame]
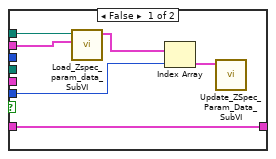
[diagram p9: hidden frame]
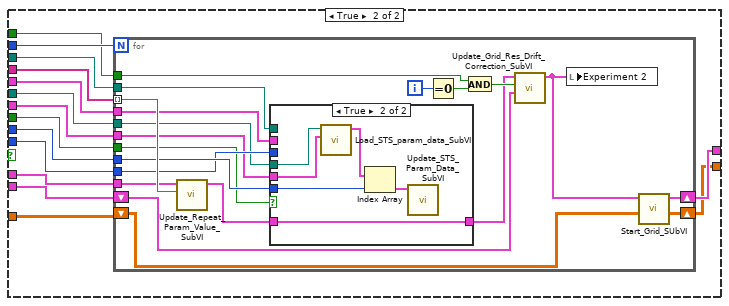
[diagram p10: hidden frame]
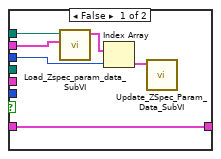
[diagram p11: hidden frame]
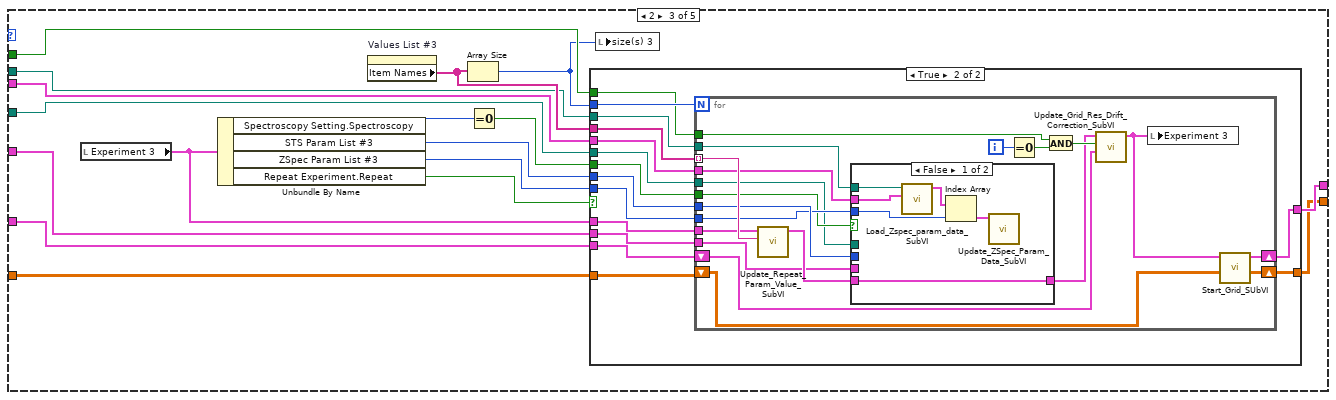
[diagram p12: hidden frame]
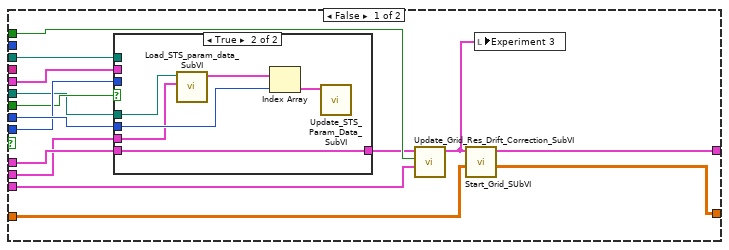
[diagram p13: hidden frame]
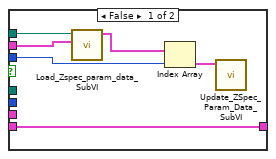
[diagram p14: hidden frame]
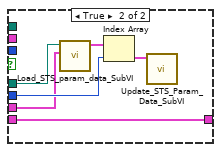
[diagram p15: hidden frame]
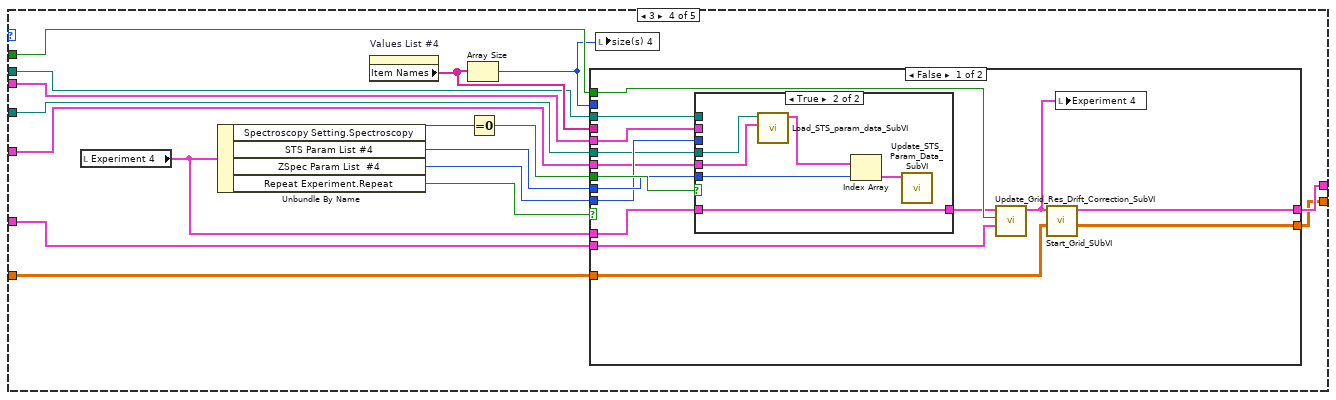
[diagram p16: hidden frame]
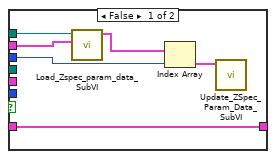
[diagram p17: hidden frame]
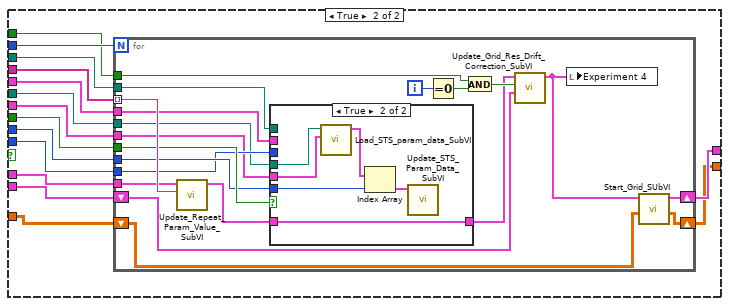
[diagram p18: hidden frame]
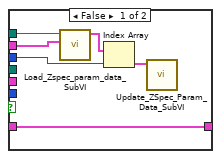
[diagram p19: hidden frame]
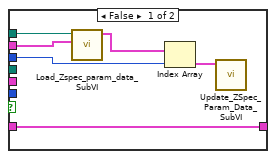
[diagram p20: hidden frame]
diagram:
  n1 = while {
    tunnel: [w12] -> w1
    stop <- w12 stop-if-true
    n2 = event shown="[1] \"START EXPERIMENT\": Value Change" {
      selector: _ -> [_ _ _ _]
      dyn-events: _ -> [_ _ _ _]
      timeout: _ -> [_ _ _ _]
      tunnel: [_ w17 _ "stop"] -> w12
      event "Duplicate Page 1": Value Change {
        n3 = event-data() -> ()  [unwired: 1 in, 4 out]
        n4 = local read "Experiment 1"() -> (w14:T4)
        n5 = property on="Experiment 3" class="Clust (strict)"("Value"=w14) -> ()  [unwired: 2 in, 2 out]
        n6 = property on="Experiment 4" class="Clust (strict)"("Value"=w14) -> ()  [unwired: 2 in, 2 out]
        n7 = property on="Experiment 5" class="Clust (strict)"("Value"=w14) -> ()  [unwired: 2 in, 2 out]
        n8 = property on="Experiment 2" class="Clust (strict)"("Value"=w14) -> ()  [unwired: 2 in, 2 out]
      }
      event "START EXPERIMENT": Value Change {
        n9 = event-data() -> ()  [unwired: 1 in, 4 out]
        n10 = local read "No. of Exp"() -> (w16:dbl)
        n11 = for {
          N: w16 -> [_]
          shift-right: [w25] -> _
          shift-left: _ -> [w27]
          tunnel: [TRUE] -> w17
          shift-right: [w19] -> _
          shift-left: dbl[][][] [] ("DC images out") -> [w18]
          i -> [w20]
          n12 = local read "Zspecparam.txt location"() -> (w24:path)
          n13 = local read "STSparam.txt location"() -> (w23:path)
          n14 = local read "data\n\n 5"() -> (w21:T1)
          n15 = local read "data\n\n 2"() -> (w22:T2)
          n16 = local write "Tab Control"(w20) -> ()
          n17 = Equal To 0?(x=w20) -> (x = 0?=w26:bool)
          n18 = case shown="4" w20 {
            tunnel: [w45 w136 w220 w318 w409] -> w25
            tunnel: w27 -> [w39 w130 w223 w315 w408]
            tunnel: w26 -> [w38 w129 w224 w316 w407]
            tunnel: w24 -> [w34 w123 w214 w308 w398]
            tunnel: w23 -> [w35 w124 w215 w307 w399]
            tunnel: w22 -> [w33 w125 w216 w306 w397]
            tunnel: w21 -> [w32 w126 w217 w305 w396]
            tunnel: [w30 w121 w212 w303 w394] -> w19
            tunnel: w18 -> [w29 w120 w211 w302 w393]
            frame 0, Default {
              n19 = local read "Experiment 1"() -> (w42:T4)
              n20 = Unbundle By Name(w42) -> ("Spectroscopy Setting.Spectroscopy"=w43:u16, "STS Param List #1"=w41:u16, "ZSpec Param List #1"=w40:u16, "Repeat Experiment.Repeat"=w36:bool)
              n21 = property on="Values List #1" class="LstBox (strict)"() -> ("Item Names"=w37:string[])  [unwired: 2 in, 2 out]
              n22 = Array Size(array=w37) -> (size(s)=w31:i32)
              n23 = Equal To 0?(x=w43) -> (x = 0?=w44:bool)
              n24 = case shown="True" w36 {
                tunnel: w31 -> [_ w87]
                tunnel: w42 -> [w56 w86]
                tunnel: w44 -> [w53 w85]
                tunnel: w41 -> [w57 w84]
                tunnel: w40 -> [w54 w83]
                tunnel: [w60 w82] -> w45
                tunnel: w39 -> [w59 w81]
                tunnel: w38 -> [w58 w80]
                tunnel: w37 -> [_ w79]
                tunnel: w35 -> [w50 w78]
                tunnel: w34 -> [w51 w77]
                tunnel: w33 -> [w49 w76]
                tunnel: w32 -> [w52 w75]
                tunnel: [w47 w74] -> w30
                tunnel: w29 -> [w46 w73]
                frame False {
                  n25 = case shown="True" w53 {
                    tunnel: w57 -> [_ w71]
                    tunnel: w49 -> [_ w70]
                    tunnel: w50 -> [_ w69]
                    tunnel: w56 -> [w63 w67]
                    tunnel: [w63 w67] -> w55
                    tunnel: w52 -> [w65 _]
                    tunnel: w51 -> [w64 _]
                    tunnel: w54 -> [w61 _]
                    frame False {
                      n26 = call "Load_Zspec_param_data_SubVI.vi"("data\n\n 5"=w65, "Zspecparam.txt location"=w64) -> ("data"=w62:T1)  [unwired: 9 in]
                      n27 = Index Array(array=w62, index=w61) -> (element=w66:T9)
                      n28 = call "Update_ZSpec_Param_Data_SubVI.vi"("output cluster"=w66) -> ()  [unwired: 11 in]
                    }
                    frame True {
                      n29 = call "Load_STS_param_data_SubVI.vi"("data\n\n in"=w70, "STSparam.txt location"=w69) -> ("data\n\n out"=w68:T2)  [unwired: 9 in]
                      n30 = Index Array(array=w68, index=w71) -> (element=w72:T10)
                      n31 = call "Update_STS_Param_Data_SubVI.vi"("STSparameters"=w72) -> ()  [unwired: 11 in]
                    }
                  }
                  n32 = call "Update_Grid_Res_Drift_Correction_SubVI.vi"("Drift Correction Settings"=w59, "Boolean"=w58, "Experiment 6"=w55) -> ("Experiment 5"=w48:T8)  [unwired: 8 in]
                  n33 = call "Start_Grid_SUbVI.vi"("DC images in"=w46, "Experiment 5"=w48) -> ("DC images out"=w47:dbl[][][], "Drift Correction Settings"=w60:T11)  [unwired: 8 in]
                  n34 = local write "Experiment 1"(w48) -> ()
                }
                frame True {
                  n35 = for {
                    N: w87 -> [_]
                    tunnel: w79 -> [w107] mode=indexing
                    tunnel: w86 -> [w106]
                    tunnel: w85 -> [w95]
                    tunnel: w84 -> [w97]
                    tunnel: w83 -> [w96]
                    shift-right: [w101] -> w82
                    shift-left: w81 -> [w105]
                    tunnel: w80 -> [w100]
                    tunnel: w78 -> [w94]
                    tunnel: w77 -> [w93]
                    tunnel: w76 -> [w92]
                    tunnel: w75 -> [w91]
                    shift-right: [w89] -> w74
                    shift-left: w73 -> [w88]
                    i -> [w104]
                    n36 = call "Update_Repeat_Param_Value_SubVI.vi"("String"=w107, "Experiment 6"=w106) -> ("Experiment 5"=w98:T8)  [unwired: 9 in]
                    n37 = case shown="True" w95 {
                      tunnel: w97 -> [_ w118]
                      tunnel: w92 -> [_ w117]
                      tunnel: w94 -> [_ w116]
                      tunnel: w98 -> [w110 w115]
                      tunnel: [w110 w115] -> w99
                      tunnel: w91 -> [w112 _]
                      tunnel: w93 -> [w111 _]
                      tunnel: w96 -> [w108 _]
                      frame False {
                        n38 = call "Load_Zspec_param_data_SubVI.vi"("data\n\n 5"=w112, "Zspecparam.txt location"=w111) -> ("data"=w109:T1)  [unwired: 9 in]
                        n39 = Index Array(array=w109, index=w108) -> (element=w113:T9)
                        n40 = call "Update_ZSpec_Param_Data_SubVI.vi"("output cluster"=w113) -> ()  [unwired: 11 in]
                      }
                      frame True {
                        n41 = call "Load_STS_param_data_SubVI.vi"("data\n\n in"=w117, "STSparam.txt location"=w116) -> ("data\n\n out"=w114:T2)  [unwired: 9 in]
                        n42 = Index Array(array=w114, index=w118) -> (element=w119:T10)
                        n43 = call "Update_STS_Param_Data_SubVI.vi"("STSparameters"=w119) -> ()  [unwired: 11 in]
                      }
                    }
                    n44 = Equal To 0?(x=w104) -> (x = 0?=w103:bool)
                    n45 = And(x=w100, y=w103) -> (x .and. y?=w102:bool)
                    n46 = call "Update_Grid_Res_Drift_Correction_SubVI.vi"("Drift Correction Settings"=w105, "Boolean"=w102, "Experiment 6"=w99) -> ("Experiment 5"=w90:T8)  [unwired: 8 in]
                    n47 = local write "Experiment 1"(w90) -> ()
                    n48 = call "Start_Grid_SUbVI.vi"("DC images in"=w88, "Experiment 5"=w90) -> ("DC images out"=w89:dbl[][][], "Drift Correction Settings"=w101:T11)  [unwired: 8 in]
                  }
                }
              }
              n49 = local write "size(s)"(w31) -> ()
            }
            frame 1 {
              n50 = local read "Experiment 2"() -> (w128:T5)
              n51 = Unbundle By Name(w128) -> ("Spectroscopy Setting.Spectroscopy"=w135:u16, "STS Param List #2"=w133:u16, "ZSpec Param List  #2"=w132:u16, "Repeat Experiment.Repeat"=w131:bool)
              n52 = property on="Values List #2" class="LstBox (strict)"() -> ("Item Names"=w127:string[])  [unwired: 2 in, 2 out]
              n53 = Array Size(array=w127) -> (size(s)=w122:i32)
              n54 = Equal To 0?(x=w135) -> (x = 0?=w134:bool)
              n55 = case shown="False" w131 {
                tunnel: w122 -> [_ w178]
                tunnel: w128 -> [w146 w177]
                tunnel: w134 -> [w148 w176]
                tunnel: w133 -> [w147 w175]
                tunnel: w132 -> [w144 w174]
                tunnel: [w151 w173] -> w136
                tunnel: w130 -> [w150 w172]
                tunnel: w129 -> [w149 w171]
                tunnel: w127 -> [_ w170]
                tunnel: w126 -> [w140 w169]
                tunnel: w125 -> [w141 w168]
                tunnel: w124 -> [w143 w167]
                tunnel: w123 -> [w142 w166]
                tunnel: [w138 w165] -> w121
                tunnel: w120 -> [w137 w164]
                frame False {
                  n56 = case shown="True" w148 {
                    tunnel: w147 -> [_ w158]
                    tunnel: w141 -> [_ w162]
                    tunnel: w143 -> [_ w161]
                    tunnel: w146 -> [w154 w159]
                    tunnel: [w154 w159] -> w145
                    tunnel: w140 -> [w156 _]
                    tunnel: w142 -> [w155 _]
                    tunnel: w144 -> [w152 _]
                    frame False {
                      n57 = call "Load_Zspec_param_data_SubVI.vi"("data\n\n 5"=w156, "Zspecparam.txt location"=w155) -> ("data"=w153:T1)  [unwired: 9 in]
                      n58 = Index Array(array=w153, index=w152) -> (element=w157:T9)
                      n59 = call "Update_ZSpec_Param_Data_SubVI.vi"("output cluster"=w157) -> ()  [unwired: 11 in]
                    }
                    frame True {
                      n60 = call "Load_STS_param_data_SubVI.vi"("data\n\n in"=w162, "STSparam.txt location"=w161) -> ("data\n\n out"=w160:T2)  [unwired: 9 in]
                      n61 = Index Array(array=w160, index=w158) -> (element=w163:T10)
                      n62 = call "Update_STS_Param_Data_SubVI.vi"("STSparameters"=w163) -> ()  [unwired: 11 in]
                    }
                  }
                  n63 = call "Update_Grid_Res_Drift_Correction_SubVI.vi"("Drift Correction Settings"=w150, "Boolean"=w149, "Experiment 6"=w145) -> ("Experiment 5"=w139:T8)  [unwired: 8 in]
                  n64 = call "Start_Grid_SUbVI.vi"("DC images in"=w137, "Experiment 5"=w139) -> ("DC images out"=w138:dbl[][][], "Drift Correction Settings"=w151:T11)  [unwired: 8 in]
                  n65 = local write "Experiment 2"(w139) -> ()
                }
                frame True {
                  n66 = for {
                    N: w178 -> [_]
                    tunnel: w170 -> [w198] mode=indexing
                    tunnel: w177 -> [w197]
                    tunnel: w176 -> [w188]
                    tunnel: w175 -> [w190]
                    tunnel: w174 -> [w189]
                    shift-right: [w192] -> w173
                    shift-left: w172 -> [w196]
                    tunnel: w171 -> [w191]
                    tunnel: w169 -> [w185]
                    tunnel: w168 -> [w184]
                    tunnel: w167 -> [w183]
                    tunnel: w166 -> [w182]
                    shift-right: [w180] -> w165
                    shift-left: w164 -> [w179]
                    i -> [w195]
                    n67 = call "Update_Repeat_Param_Value_SubVI.vi"("String"=w198, "Experiment 6"=w197) -> ("Experiment 5"=w187:T8)  [unwired: 9 in]
                    n68 = case shown="True" w188 {
                      tunnel: w190 -> [_ w209]
                      tunnel: w184 -> [_ w208]
                      tunnel: w183 -> [_ w207]
                      tunnel: w187 -> [w201 w206]
                      tunnel: [w201 w206] -> w186
                      tunnel: w185 -> [w203 _]
                      tunnel: w182 -> [w202 _]
                      tunnel: w189 -> [w199 _]
                      frame False {
                        n69 = call "Load_Zspec_param_data_SubVI.vi"("data\n\n 5"=w203, "Zspecparam.txt location"=w202) -> ("data"=w200:T1)  [unwired: 9 in]
                        n70 = Index Array(array=w200, index=w199) -> (element=w204:T9)
                        n71 = call "Update_ZSpec_Param_Data_SubVI.vi"("output cluster"=w204) -> ()  [unwired: 11 in]
                      }
                      frame True {
                        n72 = call "Load_STS_param_data_SubVI.vi"("data\n\n in"=w208, "STSparam.txt location"=w207) -> ("data\n\n out"=w205:T2)  [unwired: 9 in]
                        n73 = Index Array(array=w205, index=w209) -> (element=w210:T10)
                        n74 = call "Update_STS_Param_Data_SubVI.vi"("STSparameters"=w210) -> ()  [unwired: 11 in]
                      }
                    }
                    n75 = Equal To 0?(x=w195) -> (x = 0?=w194:bool)
                    n76 = And(x=w191, y=w194) -> (x .and. y?=w193:bool)
                    n77 = call "Update_Grid_Res_Drift_Correction_SubVI.vi"("Drift Correction Settings"=w196, "Boolean"=w193, "Experiment 6"=w186) -> ("Experiment 5"=w181:T8)  [unwired: 8 in]
                    n78 = local write "Experiment 2"(w181) -> ()
                    n79 = call "Start_Grid_SUbVI.vi"("DC images in"=w179, "Experiment 5"=w181) -> ("DC images out"=w180:dbl[][][], "Drift Correction Settings"=w192:T11)  [unwired: 8 in]
                  }
                }
              }
              n80 = local write "size(s) 2"(w122) -> ()
            }
            frame 2 {
              n81 = local read "Experiment 3"() -> (w221:T6)
              n82 = Unbundle By Name(w221) -> ("Spectroscopy Setting.Spectroscopy"=w218:u16, "STS Param List #3"=w227:u16, "ZSpec Param List #3"=w226:u16, "Repeat Experiment.Repeat"=w225:bool)
              n83 = property on="Values List #3" class="LstBox (strict)"() -> ("Item Names"=w222:string[])  [unwired: 2 in, 2 out]
              n84 = Array Size(array=w222) -> (size(s)=w213:i32)
              n85 = Equal To 0?(x=w218) -> (x = 0?=w219:bool)
              n86 = case shown="True" w225 {
                tunnel: w213 -> [_ w269]
                tunnel: w221 -> [w238 w268]
                tunnel: w219 -> [w235 w267]
                tunnel: w227 -> [w237 w266]
                tunnel: w226 -> [w236 w265]
                tunnel: [w240 w264] -> w220
                tunnel: w223 -> [w242 w263]
                tunnel: w224 -> [w241 w262]
                tunnel: w222 -> [_ w261]
                tunnel: w217 -> [w234 w257]
                tunnel: w216 -> [w233 w260]
                tunnel: w215 -> [w232 w258]
                tunnel: w214 -> [w231 w259]
                tunnel: [w229 w256] -> w212
                tunnel: w211 -> [w228 w255]
                frame False {
                  n87 = case shown="True" w235 {
                    tunnel: w237 -> [_ w253]
                    tunnel: w233 -> [_ w252]
                    tunnel: w232 -> [_ w251]
                    tunnel: w238 -> [w245 w250]
                    tunnel: [w245 w250] -> w239
                    tunnel: w234 -> [w247 _]
                    tunnel: w231 -> [w246 _]
                    tunnel: w236 -> [w243 _]
                    frame False {
                      n88 = call "Load_Zspec_param_data_SubVI.vi"("data\n\n 5"=w247, "Zspecparam.txt location"=w246) -> ("data"=w244:T1)  [unwired: 9 in]
                      n89 = Index Array(array=w244, index=w243) -> (element=w248:T9)
                      n90 = call "Update_ZSpec_Param_Data_SubVI.vi"("output cluster"=w248) -> ()  [unwired: 11 in]
                    }
                    frame True {
                      n91 = call "Load_STS_param_data_SubVI.vi"("data\n\n in"=w252, "STSparam.txt location"=w251) -> ("data\n\n out"=w249:T2)  [unwired: 9 in]
                      n92 = Index Array(array=w249, index=w253) -> (element=w254:T10)
                      n93 = call "Update_STS_Param_Data_SubVI.vi"("STSparameters"=w254) -> ()  [unwired: 11 in]
                    }
                  }
                  n94 = call "Update_Grid_Res_Drift_Correction_SubVI.vi"("Drift Correction Settings"=w242, "Boolean"=w241, "Experiment 6"=w239) -> ("Experiment 5"=w230:T8)  [unwired: 8 in]
                  n95 = call "Start_Grid_SUbVI.vi"("DC images in"=w228, "Experiment 5"=w230) -> ("DC images out"=w229:dbl[][][], "Drift Correction Settings"=w240:T11)  [unwired: 8 in]
                  n96 = local write "Experiment 3"(w230) -> ()
                }
                frame True {
                  n97 = for {
                    N: w269 -> [_]
                    tunnel: w261 -> [w289] mode=indexing
                    tunnel: w268 -> [w288]
                    tunnel: w267 -> [w277]
                    tunnel: w266 -> [w279]
                    tunnel: w265 -> [w278]
                    shift-right: [w283] -> w264
                    shift-left: w263 -> [w287]
                    tunnel: w262 -> [w282]
                    tunnel: w260 -> [w276]
                    tunnel: w259 -> [w275]
                    tunnel: w258 -> [w274]
                    tunnel: w257 -> [w273]
                    shift-right: [w271] -> w256
                    shift-left: w255 -> [w270]
                    i -> [w286]
                    n98 = call "Update_Repeat_Param_Value_SubVI.vi"("String"=w289, "Experiment 6"=w288) -> ("Experiment 5"=w281:T8)  [unwired: 9 in]
                    n99 = case shown="False" w277 {
                      tunnel: w279 -> [_ w300]
                      tunnel: w276 -> [_ w299]
                      tunnel: w274 -> [_ w298]
                      tunnel: w281 -> [w292 w297]
                      tunnel: [w292 w297] -> w280
                      tunnel: w273 -> [w294 _]
                      tunnel: w275 -> [w293 _]
                      tunnel: w278 -> [w290 _]
                      frame False {
                        n100 = call "Load_Zspec_param_data_SubVI.vi"("data\n\n 5"=w294, "Zspecparam.txt location"=w293) -> ("data"=w291:T1)  [unwired: 9 in]
                        n101 = Index Array(array=w291, index=w290) -> (element=w295:T9)
                        n102 = call "Update_ZSpec_Param_Data_SubVI.vi"("output cluster"=w295) -> ()  [unwired: 11 in]
                      }
                      frame True {
                        n103 = call "Load_STS_param_data_SubVI.vi"("data\n\n in"=w299, "STSparam.txt location"=w298) -> ("data\n\n out"=w296:T2)  [unwired: 9 in]
                        n104 = Index Array(array=w296, index=w300) -> (element=w301:T10)
                        n105 = call "Update_STS_Param_Data_SubVI.vi"("STSparameters"=w301) -> ()  [unwired: 11 in]
                      }
                    }
                    n106 = Equal To 0?(x=w286) -> (x = 0?=w285:bool)
                    n107 = And(x=w282, y=w285) -> (x .and. y?=w284:bool)
                    n108 = call "Update_Grid_Res_Drift_Correction_SubVI.vi"("Drift Correction Settings"=w287, "Boolean"=w284, "Experiment 6"=w280) -> ("Experiment 5"=w272:T8)  [unwired: 8 in]
                    n109 = local write "Experiment 3"(w272) -> ()
                    n110 = call "Start_Grid_SUbVI.vi"("DC images in"=w270, "Experiment 5"=w272) -> ("DC images out"=w271:dbl[][][], "Drift Correction Settings"=w283:T11)  [unwired: 8 in]
                  }
                }
              }
              n111 = local write "size(s) 3"(w213) -> ()
            }
            frame 3 {
              n112 = local read "Experiment 4"() -> (w313:T7)
              n113 = Unbundle By Name(w313) -> ("Spectroscopy Setting.Spectroscopy"=w310:u16, "STS Param List #4"=w311:u16, "ZSpec Param List  #4"=w312:u16, "Repeat Experiment.Repeat"=w317:bool)
              n114 = property on="Values List #4" class="LstBox (strict)"() -> ("Item Names"=w314:string[])  [unwired: 2 in, 2 out]
              n115 = Array Size(array=w314) -> (size(s)=w304:i32)
              n116 = Equal To 0?(x=w310) -> (x = 0?=w309:bool)
              n117 = case shown="False" w317 {
                tunnel: w304 -> [_ w360]
                tunnel: w313 -> [w329 w359]
                tunnel: w309 -> [w328 w358]
                tunnel: w311 -> [w327 w357]
                tunnel: w312 -> [w326 w356]
                tunnel: [w333 w355] -> w318
                tunnel: w315 -> [w332 w354]
                tunnel: w316 -> [w331 w353]
                tunnel: w314 -> [_ w352]
                tunnel: w308 -> [w324 w351]
                tunnel: w307 -> [w325 w350]
                tunnel: w306 -> [w323 w349]
                tunnel: w305 -> [w322 w348]
                tunnel: [w320 w347] -> w303
                tunnel: w302 -> [w319 w346]
                frame False {
                  n118 = case shown="True" w328 {
                    tunnel: w327 -> [_ w344]
                    tunnel: w323 -> [_ w343]
                    tunnel: w325 -> [_ w342]
                    tunnel: w329 -> [w336 w341]
                    tunnel: [w336 w341] -> w330
                    tunnel: w322 -> [w338 _]
                    tunnel: w324 -> [w337 _]
                    tunnel: w326 -> [w334 _]
                    frame False {
                      n119 = call "Load_Zspec_param_data_SubVI.vi"("data\n\n 5"=w338, "Zspecparam.txt location"=w337) -> ("data"=w335:T1)  [unwired: 9 in]
                      n120 = Index Array(array=w335, index=w334) -> (element=w339:T9)
                      n121 = call "Update_ZSpec_Param_Data_SubVI.vi"("output cluster"=w339) -> ()  [unwired: 11 in]
                    }
                    frame True {
                      n122 = call "Load_STS_param_data_SubVI.vi"("data\n\n in"=w343, "STSparam.txt location"=w342) -> ("data\n\n out"=w340:T2)  [unwired: 9 in]
                      n123 = Index Array(array=w340, index=w344) -> (element=w345:T10)
                      n124 = call "Update_STS_Param_Data_SubVI.vi"("STSparameters"=w345) -> ()  [unwired: 11 in]
                    }
                  }
                  n125 = call "Update_Grid_Res_Drift_Correction_SubVI.vi"("Drift Correction Settings"=w332, "Boolean"=w331, "Experiment 6"=w330) -> ("Experiment 5"=w321:T8)  [unwired: 8 in]
                  n126 = call "Start_Grid_SUbVI.vi"("DC images in"=w319, "Experiment 5"=w321) -> ("DC images out"=w320:dbl[][][], "Drift Correction Settings"=w333:T11)  [unwired: 8 in]
                  n127 = local write "Experiment 4"(w321) -> ()
                }
                frame True {
                  n128 = for {
                    N: w360 -> [_]
                    tunnel: w352 -> [w380] mode=indexing
                    tunnel: w359 -> [w379]
                    tunnel: w358 -> [w370]
                    tunnel: w357 -> [w369]
                    tunnel: w356 -> [w368]
                    shift-right: [w374] -> w355
                    shift-left: w354 -> [w378]
                    tunnel: w353 -> [w373]
                    tunnel: w351 -> [w367]
                    tunnel: w350 -> [w366]
                    tunnel: w349 -> [w365]
                    tunnel: w348 -> [w364]
                    shift-right: [w362] -> w347
                    shift-left: w346 -> [w361]
                    i -> [w377]
                    n129 = call "Update_Repeat_Param_Value_SubVI.vi"("String"=w380, "Experiment 6"=w379) -> ("Experiment 5"=w372:T8)  [unwired: 9 in]
                    n130 = case shown="True" w370 {
                      tunnel: w369 -> [_ w391]
                      tunnel: w365 -> [_ w390]
                      tunnel: w366 -> [_ w389]
                      tunnel: w372 -> [w381 w387]
                      tunnel: w364 -> [w385 _]
                      tunnel: w367 -> [w384 _]
                      tunnel: w368 -> [w382 _]
                      tunnel: [w381 w387] -> w371
                      frame False {
                        n131 = call "Load_Zspec_param_data_SubVI.vi"("data\n\n 5"=w385, "Zspecparam.txt location"=w384) -> ("data"=w383:T1)  [unwired: 9 in]
                        n132 = Index Array(array=w383, index=w382) -> (element=w386:T9)
                        n133 = call "Update_ZSpec_Param_Data_SubVI.vi"("output cluster"=w386) -> ()  [unwired: 11 in]
                      }
                      frame True {
                        n134 = call "Load_STS_param_data_SubVI.vi"("data\n\n in"=w390, "STSparam.txt location"=w389) -> ("data\n\n out"=w388:T2)  [unwired: 9 in]
                        n135 = Index Array(array=w388, index=w391) -> (element=w392:T10)
                        n136 = call "Update_STS_Param_Data_SubVI.vi"("STSparameters"=w392) -> ()  [unwired: 11 in]
                      }
                    }
                    n137 = Equal To 0?(x=w377) -> (x = 0?=w376:bool)
                    n138 = And(x=w373, y=w376) -> (x .and. y?=w375:bool)
                    n139 = call "Update_Grid_Res_Drift_Correction_SubVI.vi"("Drift Correction Settings"=w378, "Boolean"=w375, "Experiment 6"=w371) -> ("Experiment 5"=w363:T8)  [unwired: 8 in]
                    n140 = local write "Experiment 4"(w363) -> ()
                    n141 = call "Start_Grid_SUbVI.vi"("DC images in"=w361, "Experiment 5"=w363) -> ("DC images out"=w362:dbl[][][], "Drift Correction Settings"=w374:T11)  [unwired: 8 in]
                  }
                }
              }
              n142 = local write "size(s) 4"(w304) -> ()
            }
            frame 4 {
              n143 = local read "Experiment 5"() -> (w404:T8)
              n144 = Unbundle By Name(w404) -> ("Spectroscopy Setting.Spectroscopy"=w400:u16, "STS Param List #5"=w402:u16, "ZSpec Param List #5"=w403:u16, "Repeat Experiment.Repeat"=w406:bool)
              n145 = property on="Values List #5" class="LstBox (strict)"() -> ("Item Names"=w405:string[])  [unwired: 2 in, 2 out]
              n146 = Array Size(array=w405) -> (size(s)=w395:i32)
              n147 = Equal To 0?(x=w400) -> (x = 0?=w401:bool)
              n148 = case shown="False" w406 {
                selector: w406 -> [w419 _]
                tunnel: w395 -> [_ w451]
                tunnel: w404 -> [w417 w450]
                tunnel: w401 -> [_ w449]
                tunnel: w402 -> [w420 w448]
                tunnel: w403 -> [w421 w447]
                tunnel: [w424 w446] -> w409
                tunnel: w408 -> [w423 w445]
                tunnel: w407 -> [w422 w444]
                tunnel: w405 -> [_ w443]
                tunnel: w399 -> [w416 w442]
                tunnel: w398 -> [w415 w441]
                tunnel: w397 -> [w414 w440]
                tunnel: w396 -> [w413 w439]
                tunnel: [w411 w438] -> w394
                tunnel: w393 -> [w410 w437]
                frame False {
                  n149 = case shown="True" w419 {
                    tunnel: w420 -> [_ w435]
                    tunnel: w414 -> [_ w434]
                    tunnel: w416 -> [_ w433]
                    tunnel: w417 -> [w427 w431]
                    tunnel: [w427 w431] -> w418
                    tunnel: w413 -> [w429 _]
                    tunnel: w415 -> [w428 _]
                    tunnel: w421 -> [w425 _]
                    frame False {
                      n150 = call "Load_Zspec_param_data_SubVI.vi"("data\n\n 5"=w429, "Zspecparam.txt location"=w428) -> ("data"=w426:T1)  [unwired: 9 in]
                      n151 = Index Array(array=w426, index=w425) -> (element=w430:T9)
                      n152 = call "Update_ZSpec_Param_Data_SubVI.vi"("output cluster"=w430) -> ()  [unwired: 11 in]
                    }
                    frame True {
                      n153 = call "Load_STS_param_data_SubVI.vi"("data\n\n in"=w434, "STSparam.txt location"=w433) -> ("data\n\n out"=w432:T2)  [unwired: 9 in]
                      n154 = Index Array(array=w432, index=w435) -> (element=w436:T10)
                      n155 = call "Update_STS_Param_Data_SubVI.vi"("STSparameters"=w436) -> ()  [unwired: 11 in]
                    }
                  }
                  n156 = call "Update_Grid_Res_Drift_Correction_SubVI.vi"("Drift Correction Settings"=w423, "Boolean"=w422, "Experiment 6"=w418) -> ("Experiment 5"=w412:T8)  [unwired: 8 in]
                  n157 = call "Start_Grid_SUbVI.vi"("DC images in"=w410, "Experiment 5"=w412) -> ("DC images out"=w411:dbl[][][], "Drift Correction Settings"=w424:T11)  [unwired: 8 in]
                  n158 = local write "Experiment 5"(w412) -> ()
                }
                frame True {
                  n159 = for {
                    N: w451 -> [_]
                    tunnel: w443 -> [w471] mode=indexing
                    tunnel: w450 -> [w470]
                    tunnel: w449 -> [w459]
                    tunnel: w448 -> [w460]
                    tunnel: w447 -> [w461]
                    shift-right: [w465] -> w446
                    shift-left: w445 -> [w469]
                    tunnel: w444 -> [w464]
                    tunnel: w442 -> [w458]
                    tunnel: w441 -> [w457]
                    tunnel: w440 -> [w456]
                    tunnel: w439 -> [w455]
                    shift-right: [w453] -> w438
                    shift-left: w437 -> [w452]
                    i -> [w468]
                    n160 = call "Update_Repeat_Param_Value_SubVI.vi"("String"=w471, "Experiment 6"=w470) -> ("Experiment 5"=w463:T8)  [unwired: 9 in]
                    n161 = case shown="True" w459 {
                      tunnel: w460 -> [_ w482]
                      tunnel: w456 -> [_ w481]
                      tunnel: w458 -> [_ w480]
                      tunnel: w463 -> [w474 w479]
                      tunnel: [w474 w479] -> w462
                      tunnel: w455 -> [w476 _]
                      tunnel: w457 -> [w475 _]
                      tunnel: w461 -> [w472 _]
                      frame False {
                        n162 = call "Load_Zspec_param_data_SubVI.vi"("data\n\n 5"=w476, "Zspecparam.txt location"=w475) -> ("data"=w473:T1)  [unwired: 9 in]
                        n163 = Index Array(array=w473, index=w472) -> (element=w477:T9)
                        n164 = call "Update_ZSpec_Param_Data_SubVI.vi"("output cluster"=w477) -> ()  [unwired: 11 in]
                      }
                      frame True {
                        n165 = call "Load_STS_param_data_SubVI.vi"("data\n\n in"=w481, "STSparam.txt location"=w480) -> ("data\n\n out"=w478:T2)  [unwired: 9 in]
                        n166 = Index Array(array=w478, index=w482) -> (element=w483:T10)
                        n167 = call "Update_STS_Param_Data_SubVI.vi"("STSparameters"=w483) -> ()  [unwired: 11 in]
                      }
                    }
                    n168 = Equal To 0?(x=w468) -> (x = 0?=w467:bool)
                    n169 = And(x=w464, y=w467) -> (x .and. y?=w466:bool)
                    n170 = call "Update_Grid_Res_Drift_Correction_SubVI.vi"("Drift Correction Settings"=w469, "Boolean"=w466, "Experiment 6"=w462) -> ("Experiment 5"=w454:T8)  [unwired: 8 in]
                    n171 = local write "Experiment 5"(w454) -> ()
                    n172 = call "Start_Grid_SUbVI.vi"("DC images in"=w452, "Experiment 5"=w454) -> ("DC images out"=w453:dbl[][][], "Drift Correction Settings"=w465:T11)  [unwired: 8 in]
                  }
                }
              }
              n173 = local write "size(s) 5"(w395) -> ()
            }
          }
        }
      }
      event "Update STS/Zspec Param List": Value Change {
        n174 = event-data() -> ()  [unwired: 1 in, 6 out]
        n175 = local read "STSparam.txt location"() -> (w490:path)
        n176 = local read "Zspecparam.txt location"() -> (w489:path)
        n177 = control-ref of="data\n\n 2"() -> (w488:refnum<vi>)
        n178 = call "Load_STS_param_options_SubVI.vi"("STSparam.txt location"=w490, "Array in"=w488) -> ("error out"=w491:errorcluster, "Array"=w485:string[])  [unwired: 8 in]
        n179 = control-ref of="data\n\n 5"() -> (w487:refnum<vi>)
        n180 = call "Load_Zspec_param_options_SubVI.vi"("error in (no error)"=w491, "Zspecparam.txt location"=w489, "Array in"=w487) -> ("Array"=w486:string[])  [unwired: 8 in]
        n181 = for {
          N: 5 -> [_]
          tunnel: w486 -> [w493]
          tunnel: w485 -> [w492]
          i -> [w494]
          n182 = case shown="0, Default" w494 {
            tunnel: w493 -> [w496 w498 w500 w502 w504]
            tunnel: w492 -> [w495 w497 w499 w501 w503]
            frame 0, Default {
              n183 = property on="STS Param List #1" class="Ring (strict)"("Strings []"=w495) -> ()  [unwired: 2 in, 2 out]
              n184 = property on="ZSpec Param List #1" class="Ring (strict)"("Strings []"=w496) -> ()  [unwired: 2 in, 2 out]
            }
            frame 1 {
              n185 = property on="STS Param List #2" class="Ring (strict)"("Strings []"=w497) -> ()  [unwired: 2 in, 2 out]
              n186 = property on="ZSpec Param List  #2" class="Ring (strict)"("Strings []"=w498) -> ()  [unwired: 2 in, 2 out]
            }
            frame 2 {
              n187 = property on="STS Param List #3" class="Ring (strict)"("Strings []"=w499) -> ()  [unwired: 2 in, 2 out]
              n188 = property on="ZSpec Param List #3" class="Ring (strict)"("Strings []"=w500) -> ()  [unwired: 2 in, 2 out]
            }
            frame 3 {
              n189 = property on="STS Param List #4" class="Ring (strict)"("Strings []"=w501) -> ()  [unwired: 2 in, 2 out]
              n190 = property on="ZSpec Param List  #4" class="Ring (strict)"("Strings []"=w502) -> ()  [unwired: 2 in, 2 out]
            }
            frame 4 {
              n191 = property on="STS Param List #5" class="Ring (strict)"("Strings []"=w503) -> ()  [unwired: 2 in, 2 out]
              n192 = property on="ZSpec Param List #5" class="Ring (strict)"("Strings []"=w504) -> ()  [unwired: 2 in, 2 out]
            }
          }
        }
      }
      event "stop": Value Change {
        n193 = event-data() -> ()  [unwired: 1 in, 4 out]
      }
    }
    n194 = property on="Values List #4" class="LstBox (strict)"() -> ("Item Names"=w3:string[])  [unwired: 2 in, 2 out]
    n195 = property on="Values List #1" class="LstBox (strict)"() -> ("Item Names"=w6:string[])  [unwired: 2 in, 2 out]
    n196 = property on="Values List #5" class="LstBox (strict)"() -> ("Item Names"=w2:string[])  [unwired: 2 in, 2 out]
    n197 = property on="Values List #2" class="LstBox (strict)"() -> ("Item Names"=w5:string[])  [unwired: 2 in, 2 out]
    n198 = Wait (ms)(milliseconds to wait=u32 100) -> ()  [unwired: 1 out]
    n199 = Array Size(array=w3) -> (size(s)=w8:i32)
    n200 = Array Size(array=w6) -> (size(s)=w11:i32)
    n201 = Array Size(array=w2) -> (size(s)=w7:i32)
    n202 = Array Size(array=w5) -> (size(s)=w10:i32)
    n203 = local write "size(s)"(w11) -> ()
    n204 = local write "size(s) 4"(w8) -> ()
    n205 = local write "size(s) 5"(w7) -> ()
    n206 = local write "size(s) 2"(w10) -> ()
    n207 = property on="Values List #3" class="LstBox (strict)"() -> ("Item Names"=w4:string[])  [unwired: 2 in, 2 out]
    n208 = Array Size(array=w4) -> (size(s)=w9:i32)
    n209 = local write "size(s) 3"(w9) -> ()
  }
  n210 = case shown="False" w1 {
    frame False {
    }
    frame True {
      n211 = call <userlib>:"Prog Interface - OpenAppRef.vi"() -> ("Error out"=w509:errorcluster, "Application reference"=w510:refnum<vi>)  [unwired: 6 in]
      n212 = call <userlib>:"Point Erase.vi"("Application ref in"=w510, "Point index (-1=All points)"=0, "error in (no error)"=w509) -> ("Application ref out"=w506:refnum<vi>, "error out"=w507:errorcluster)  [unwired: 11 in]
      n213 = Close Reference(reference=w506, error in (no error)=w507) -> ()  [unwired: 1 out]
    }
  }
